vi "PCS-home.vi"() -> (3 "Stop":bool)   [LabVIEW 2011]
uses:
  <vilib>/Analysis/2dsp.llb/Integral Method.ctl
  <vilib>/Analysis/NI_AALPro.lvlib
  <vilib>/ptbypt/NI_PtbyPt.lvlib
  <vilib>/Analysis/NI_AALBase.lvlib
panel:
  out "Pfit":dbl
  out "Pcin":dbl(slide) scale=0.0..20.0 scale format="%#_2g"
  out "RTD-chamber (ºC)":sgl format="%0.2f"
  out "RTD-01 (ºC)":sgl format="%0.2f"
  out "RTD-02 (ºC)":sgl format="%0.2f"
  out "estado":bool
  out "slop":bool
  out "descarga 2":bool=TRUE
  out "time-loop":dbl
  in  "clear sample":bool
  out "cont_vacuo 2":u32[](array[numeric])
  out "Numeric":dbl
  out "Volume File":string
  out "Isotherm File":string
  in  "PCS":bool
  out "pathISO":path
  out "pathVV":path
  in  "Vertical Pause Button":bool
  out "tempo":dbl[](array[numeric])
  out "tempo 2":dbl[](array[numeric])
  out "output array":dbl[][](array[numeric])
  in  "T Ctrl":bool
  out "graph_completo":dynamicdata(graph)
  out "Vol02":dbl(slide) scale=0.0..20.0 scale format="%#_2g"
  out "Chamber":dbl(slide) scale=0.0..20.0 scale format="%#_2g"
  out "Vol01":dbl(slide) scale=0.0..20.0 scale format="%#_2g"
  in  "Tab Control":T1(tab)
  in  "Save As":bool
  out "path":path
  out "File name":string
  in  "Sample name":string
  in  "Nota 01":string
  in  "Open Button":bool
  out "stripped path":path
  in  "New file":string
  in  "array":dbl[](array[numeric])
  in  "SetP Array":bool
  in  "Npoint 2":i32
  in  "Pmax 2":i32
  out "Inter P 2":dbl
  out "Set ISO":dbl
  out "set P ISO":dbl
  in  "ISO Start":bool
  out "Inter P":dbl
  in  "Pmax":i32
  in  "Npoint":i32
  out "Set v v":dbl
  out "set P":dbl
  in  "V V Start":bool
  in  "Pressure Max":dbl
  in  "N cycles":dbl
  in  "Ch Max":bool
  in  "Save Discharge":bool
  out "Set ChM":dbl
  out "Cycles":dbl
  in  "Kinetic Save":bool
  out "slop01":T2(graph)
  out "fit-all":T3(graph)
  in  "SP-vol-01":dbl
  in  "command":string
  out "Abrir Gas":bool
  out "time (min)":dbl
  in  "Mininum Slope":dbl format="%#_6p"
  in  "total Time(min)":dbl
  in  "dp/dt min":dbl
  out "dp/dt":dbl format="%0.2f"
  out "slope":dbl format="%#_2p"
  out "time":dbl
  in  "t-vacuo (s)":dbl=1000.0
  in  "dp/dt min 2":dbl
  out "time (min) 2":dbl
  out "dp/dt 2":dbl format="%0.2f"
  in  "total Time(min) 2":dbl
  in  "Mininum Slope 2":dbl format="%#_6p"
  out "fit-all 2":T3(graph)
  out "slop01 2":T2(graph)
  out "slope 2":dbl format="%#_2p"
  out "vacuo (mBar)":dbl(knob) scale=0.0..20.0
  out "N 1bar":i32
  in  "t-vacuo (s) clean":dbl=1000.0
  out "time 3":dbl
  in  "New Button":bool
  out "Waveform T":dynamicdata(graph)
  out "ThermC":dbl(slide) scale=0.0..150.0
  in  "Ndata":i32
  in  "SP":dbl(slide) scale=0.0..150.0
  out "D-mean":dbl format="%0.2f"
  out "I-mean":dbl format="%0.2f"
  out "intrp- T":dbl format="%0.2f"
  out "min":dbl
  out "Max":dbl
  in  "PIDmin":dbl
  in  "PIDMax":dbl
  in  "PID":bool
  out "Ganho":dbl
  in  "Kp":dbl(slide) scale=0.0..10.0
  in  "D (Td)":bool
  in  "Kd(s)":dbl(slide) scale=0.0..10.0
  in  "I (Ti)":bool
  in  "Ki(s)":dbl(slide) scale=0.0..10.0
  out "milisec":dbl
  in  "fator Ganho":dbl=1.0
  out "t-on":dbl
  out "t-PID":bool
  in  "time (s) Loop":dbl
  in  "T - ON/OFF":bool
  in  "PID-ON/OFF":bool
  out "PID limit":bool
  in  "PID limit 2":dbl
  out "pause":bool
  in  "X time Off":dbl
  out "milisec 2":dbl
  out "ON/OFF":bool
  in  "close All":bool
  out "cont_desc":dbl[](array[numeric])
  out "Pvol2":dbl[](array[numeric])
  out "time 2":dbl[](array[numeric])
  out "cont_desc min":dbl[](array[numeric])
  out "Pvol2 total":dbl[](array[numeric])
  out "time (min) 3":dbl[](array[numeric])
  out "dP/dt":dbl[](array[numeric])
  out "x >= y? 2":bool
  out "cont_vacuo":u32[](array[numeric])
  out "PCv1":dbl[](array[numeric])
  out "t carga":dbl[](array[numeric])
  out "count":u32[](array[numeric])
  out "x >= y?":bool
  out "count 2":u32[](array[numeric])
  out "t completo":dbl[](array[numeric])
  out "PCv1 completo":dbl[](array[numeric])
  out "derivada 2":dbl[](array[numeric]) format="%#_4p"
  in  "initialize":bool
  out "SlopArray":dbl[](array[numeric]) format="%#_3p"
  out "cont":dbl[](array[numeric]) format="%#_6p"
  out "size(s)":i32
  in  "cargas-vol1":dbl
  in  "Discharge":bool
  in  "Charge":bool
  in  "stop":bool
  # "PCS - Pressure cycling system"
  # "Sorption isotherm"
  # "Maximum Charge"
  # "Void Volume"
  # "PID controller"
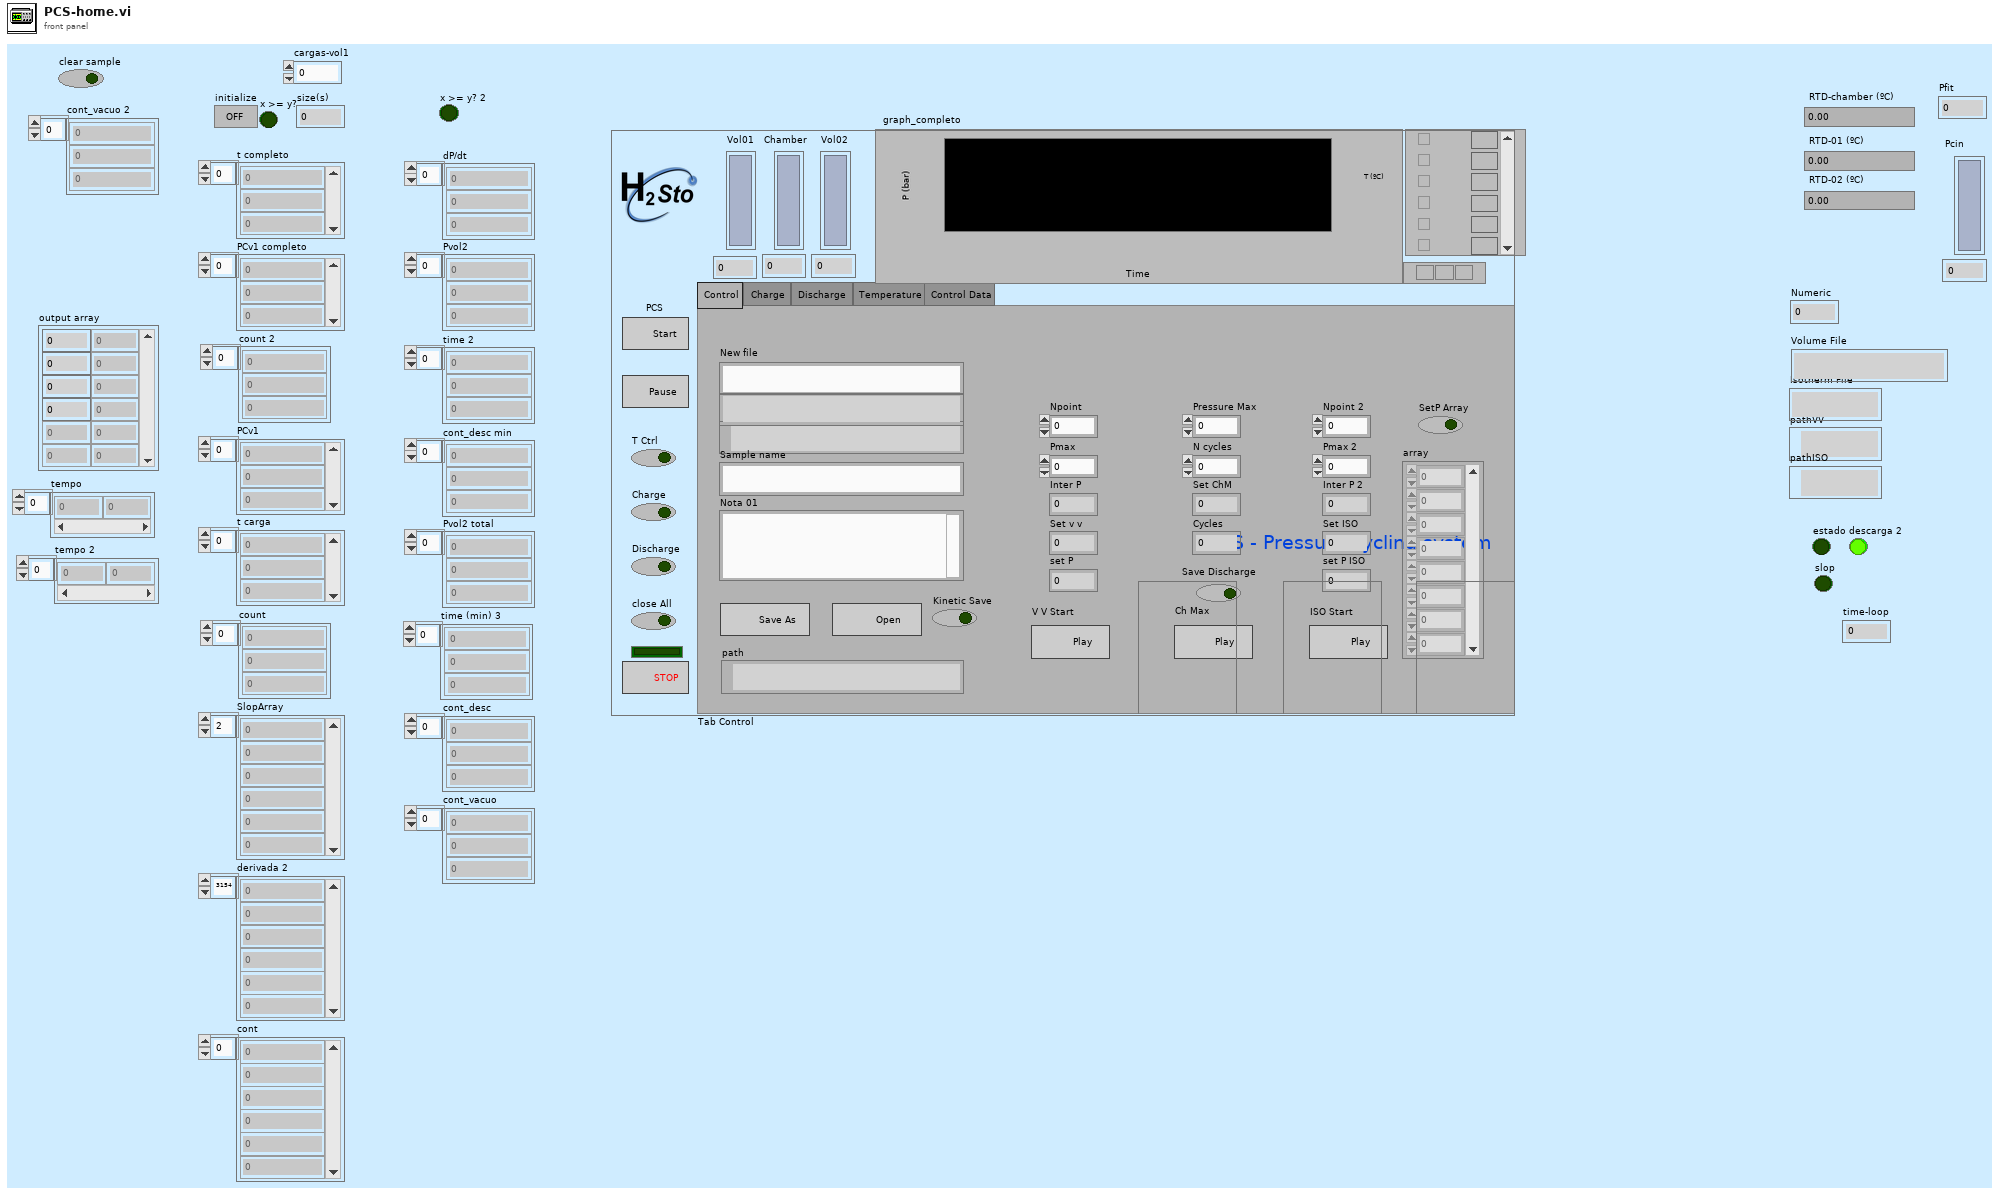
[diagram p1: front panel]
types:
  T1 = enum32{"Control", "Charge ", "Discharge ", "Temperature", "Control Data"}
  T2 = cluster{"Value":dbl[], "Best Linear Fit":dbl[]}[]
  T3 = cluster{"Value":dbl[], "Best Polynomial Fit":dbl[]}[]
  T4 = enum16{"open", "replace", "create", "open or create", "replace or create", "replace or create with confirmation"}
  T5 = enum16{"Linear", "Polynomial", "Spline", "Rational"}
  T6 = cluster{"Type of Interpolation":enum16{"Linear", "Polynomial", "Spline", "Rational"}, "Points Between":i32}
  T7 = typedef "NI_AALPro.lvlib/Integral Method.ctl" = i32
  T8 = cluster{"Value":dbl[], "Best Polynomial Fit":dbl[]}
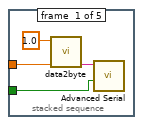
[diagram p2: hidden frame]
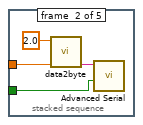
[diagram p3: hidden frame]
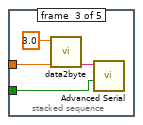
[diagram p4: hidden frame]
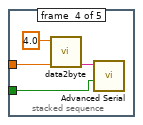
[diagram p5: hidden frame]
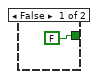
[diagram p6: hidden frame]
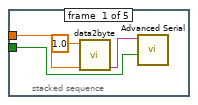
[diagram p8: hidden frame]
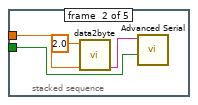
[diagram p9: hidden frame]
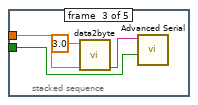
[diagram p10: hidden frame]
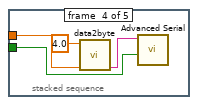
[diagram p11: hidden frame]
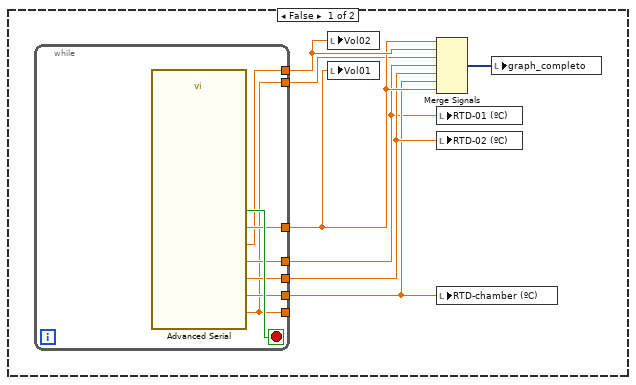
[diagram p12: hidden frame]
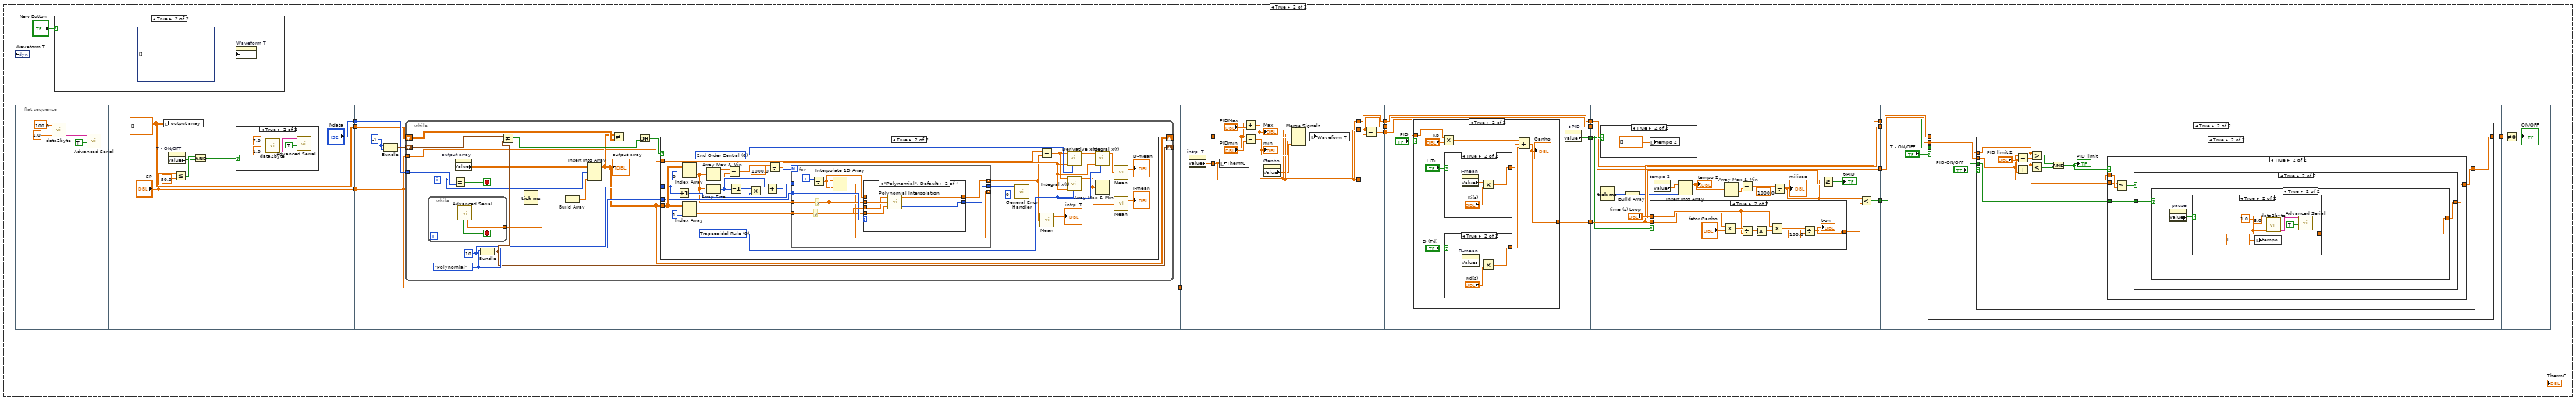
[diagram p13: hidden frame]
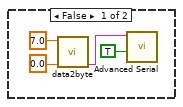
[diagram p15: hidden frame]
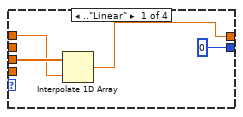
[diagram p17: hidden frame]
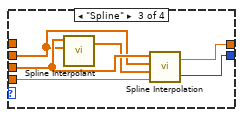
[diagram p18: hidden frame]
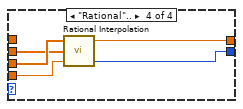
[diagram p19: hidden frame]
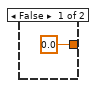
[diagram p20: hidden frame]
diagram:
  w1 = FALSE ("PCS")
  w8 = 1.0 ("Set ChM")
  n1 = while {
    stop <- w46 stop-if-true
    n2 = flat-sequence {
      tunnel: [w1623] -> w54
      tunnel: [w1622] -> w53
      tunnel: [w1618] -> w52
      tunnel: [w1621] -> w51
      tunnel: w54 -> [w1669]
      tunnel: w53 -> [w1668]
      tunnel: w52 -> [w1667]
      tunnel: w51 -> [w1659]
      frame #0 {
        n3 = case shown="True" "Save As" {
          selector: "Save As" -> [_ w1646]
          tunnel: [w1642 w1647] -> w1624
          tunnel: [FALSE w1646] -> w1623
          frame False {
            n4 = property on="path" class="Path"() -> ("Value"=w1642:path)  [unwired: 2 in, 2 out]
          }
          frame True {
            n5 = call "data_file.vi"("Nota 01"="Nota 01", "Sample name"="Sample name", "File name"="New file") -> ("path"=w1647:path)  [unwired: 8 in]
          }
        }
        n6 = local write "path"(w1624) -> ()
        n7 = Strip Path(path=w1624) -> (stripped path=w1620:path, name=w1619:string)
        "stripped path" <- w1620
        n8 = local write "File name"(w1619) -> ()
        n9 = case shown="True" "Open Button" {
          selector: "Open Button" -> [_ w1632]
          tunnel: [FALSE w1632] -> w1622
          tunnel: [w1628 w1631] -> w1621
          tunnel: w1620 -> [w1628 _]
          tunnel: [w1627 w1630] -> w1618
          tunnel: w1619 -> [w1627 _]
          frame False {
          }
          frame True {
            n10 = File Dialog(6:"*.txt" ("pattern label")) -> (0:w1636:errorcluster, 3:w1635:path)  [unwired: 3 in, 5 out]
            n11 = Open/Create/Replace File(file path (use dialog)=w1635, error in=w1636, operation (0:open)=T4."open", access (0:read/write)=enum16{"read/write", "read-only", "write-only"}."read/write") -> (refnum out=w1638:refnum<file>, error out=w1637:errorcluster)  [unwired: 2 in, 1 out]
            n12 = Close File(refnum=w1638, error in=w1637) -> (path=w1634:path)  [unwired: 1 out]
            n13 = local write "path"(w1634) -> ()
            n14 = Strip Path(path=w1634) -> (stripped path=w1631:path, name=w1630:string)
            n15 = local write "stripped path"(w1631) -> ()
            n16 = local write "File name"(w1630) -> ()
          }
        }
      }
      frame #1 {
        w1649 = "\t"
        w1661 = "\t"
        n17 = Or(x=w1669, y=w1668) -> (x .or. y?=w1670:bool)
        n18 = Concatenate Strings("set" ("search string/char (-)"), w1661, "Pv1" ("search string/char (-)"), w1661, "Pc" ("search string/char (-)"), w1661, "Tv1" ("search string/char (-)"), w1661, "Tc" ("search string/char (-)")) -> (w1651:string)
        n19 = Concatenate Strings("Cycle" ("search string/char (-)"), w1649, "set" ("search string/char (-)"), w1649, "Pit(vol1)" ("search string/char (-)"), w1649, "Pf2(Pc)" ("search string/char (-)"), w1649, "ZPf2(Pv2)" ("search string/char (-)"), w1649, "T1" ("search string/char (-)"), w1649, "Tc" ("search string/char (-)"), w1649, "T2" ("search string/char (-)")) -> (w1650:string)
        n20 = property on="path" class="Path"() -> ("Value"=w1666:path)  [unwired: 2 in, 2 out]
        n21 = case shown="True" w1670 {
          tunnel: w1667 -> [_ w1690]
          tunnel: w1659 -> [_ w1689]
          tunnel: w1666 -> [_ w1684]
          tunnel: w1651 -> [_ w1675]
          tunnel: w1650 -> [_ w1672]
          frame False {
          }
          frame True {
            n22 = flat-sequence {
              tunnel: w1689 -> [w1699]
              tunnel: w1690 -> [w1700]
              tunnel: [w1700] -> w1688
              tunnel: [w1699] -> w1687
              tunnel: w1684 -> [w1693]
              tunnel: [w1694] -> w1683
              tunnel: [w1693] -> w1681
              tunnel: w1675 -> [w1692]
              tunnel: [w1692] -> w1674
              tunnel: [w1691] -> w1673
              tunnel: w1672 -> [w1691]
              tunnel: w1688 -> [w1729]
              tunnel: w1687 -> [w1715]
              tunnel: [w1724] -> w1686
              tunnel: [w1723] -> w1685
              tunnel: w1683 -> [w1704]
              tunnel: [w1726] -> w1682
              tunnel: w1681 -> [w1725]
              tunnel: [w1725] -> w1680
              tunnel: [w1709] -> w1677
              tunnel: [w1708] -> w1676
              tunnel: w1674 -> [w1703]
              tunnel: w1673 -> [w1702]
              tunnel: [w1701] -> w1671
              tunnel: w1686 -> [w1744]
              tunnel: w1685 -> [w1743]
              tunnel: w1682 -> [w1742]
              tunnel: w1680 -> [w1741]
              tunnel: [w1741] -> w1679
              tunnel: w1677 -> [w1736]
              tunnel: w1676 -> [w1735]
              tunnel: w1671 -> [w1734]
              tunnel: w1679 -> [w1747]
              tunnel: [w1747] -> w1678
              tunnel: w1678 -> [w1767]
              frame #0 {
                n23 = Open/Create/Replace File(file path (use dialog)=w1693) -> (refnum out=w1697:refnum<file>, error out=w1698:errorcluster)  [unwired: 5 in, 1 out]
                n24 = Read from Text File(file (use dialog)=w1697, error in=w1698) -> (refnum out=w1695:refnum<file>, text=w1694:string, error out=w1696:errorcluster)  [unwired: 2 in, 1 out]
                n25 = Close File(refnum=w1695, error in=w1696) -> ()  [unwired: 2 out]
              }
              frame #1 {
                w1705 = "\r"
                w1710 = enum16{"start", "end", "current"}."end" ("from (0:start)")
                w1728 = "\r"
                w1711 = T4."replace or create with confirmation" ("operation (0:open)")
                n26 = Search/Split String(string=w1729, search string/char (-)=".txt") -> (substring before match=w1717:string, match + rest of string=w1718:string)  [unwired: 1 in, 1 out]
                n27 = Concatenate Strings(w1717, "_vv" ("search string/char (-)"), w1718) -> (w1731:string)
                "Volume File" <- w1731
                n28 = Concatenate Strings(w1717, "_iso" ("search string/char (-)"), w1718) -> (w1716:string)
                "Isotherm File" <- w1716
                n29 = Build Path(base path=w1715, name or relative path=w1731) -> (appended path=w1730:path)
                n30 = Build Path(base path=w1715, name or relative path=w1716) -> (appended path=w1712:path)
                n31 = Concatenate Strings(w1728, w1704, "============" ("search string/char (-)"), w1728, w1703, "\r\n") -> (w1726:string)
                n32 = Concatenate Strings(w1705, w1704, "============" ("search string/char (-)"), w1705, w1702, "\r\n") -> (w1701:string)
                n33 = Open/Create/Replace File(file path (use dialog)=w1730, operation (0:open)=w1711) -> (refnum out=w1722:refnum<file>, error out=w1721:errorcluster)  [unwired: 4 in, 1 out]
                n34 = Open/Create/Replace File(file path (use dialog)=w1712, operation (0:open)=w1711) -> (refnum out=w1713:refnum<file>, error out=w1714:errorcluster)  [unwired: 4 in, 1 out]
                n35 = Set File Position(refnum=w1722, from (0:start)=w1710, error in=w1721) -> (refnum out=w1724:refnum<file>, error out=w1723:errorcluster)  [unwired: 1 in]
                n36 = Set File Position(refnum=w1713, from (0:start)=w1710, error in=w1714) -> (refnum out=w1709:refnum<file>, error out=w1708:errorcluster)  [unwired: 1 in]
              }
              frame #2 {
                n37 = Write to Text File(file (use dialog)=w1744, text=w1742, error in=w1743) -> (refnum out=w1746:refnum<file>, error out=w1745:errorcluster)  [unwired: 1 in, 1 out]
                n38 = Write to Text File(file (use dialog)=w1736, text=w1734, error in=w1735) -> (refnum out=w1737:refnum<file>, error out=w1738:errorcluster)  [unwired: 1 in, 1 out]
                n39 = Close File(refnum=w1746, error in=w1745) -> (path=→"pathVV":path)  [unwired: 1 out]
                n40 = Close File(refnum=w1737, error in=w1738) -> (path=→"pathISO":path)  [unwired: 1 out]
              }
              frame #3 {
              }
              frame #4 {
                w1766 = "\t"
                n41 = Open/Create/Replace File(file path (use dialog)=w1767, access (0:read/write)=enum16{"read/write", "read-only", "write-only"}."write-only") -> (refnum out=w1755:refnum<file>, error out=w1751:errorcluster)  [unwired: 4 in, 1 out]
                n42 = Set File Position(refnum=w1755, from (0:start)=enum16{"start", "end", "current"}."end", error in=w1751) -> (refnum out=w1754:refnum<file>, error out=w1753:errorcluster)  [unwired: 1 in]
                n43 = Concatenate Strings("============" ("search string/char (-)"), "\r", "Date-time" ("search string/char (-)"), w1766, "Pv1" ("search string/char (-)"), w1766, "Pc" ("search string/char (-)"), w1766, "Pv2" ("search string/char (-)"), w1766, "T1" ("search string/char (-)"), w1766, "Tc" ("search string/char (-)"), w1766, "T2" ("search string/char (-)"), w1766, "Pcin" ("search string/char (-)"), "\r\n") -> (w1758:string)
                n44 = Write to Text File(file (use dialog)=w1754, text=w1758, error in=w1753) -> (refnum out=w1768:refnum<file>, error out=w1769:errorcluster)  [unwired: 1 in, 1 out]
                n45 = Close File(refnum=w1768, error in=w1769) -> ()  [unwired: 2 out]
              }
            }
          }
        }
      }
    }
    n46 = property class="VI"() -> (error out=w56:errorcluster, "Front Panel"=w57:refnum<vi>)  [unwired: 2 in, 1 out]
    n47 = flat-sequence {
      tunnel: [w1471] -> w45
      frame #0 {
        n48 = case shown="True" "Kinetic Save" {
          frame False {
            n49 = while {
              tunnel: [w100] -> w92
              tunnel: [w95] -> w89
              tunnel: [w99] -> w93
              tunnel: [w97] -> w88
              tunnel: [w96] -> w91
              tunnel: [w98] -> w90
              tunnel: [w95] -> _
              stop <- w101 stop-if-true
              n50 = call "Advanced Serial.vi"() -> ("RTD-02 (ºC)"=w96:sgl, "RTD-01 (ºC)"=w97:sgl, "vacuo (mBar)"=w95:dbl, "P02 (Bar)"=w99:dbl, "RTD-chamber (ºC)"=w98:sgl, "P01 (Bar)"=w100:dbl, "32bytes"=w101:bool)  [unwired: 5 in]
            }
            n51 = local write "Vol02"(w93) -> ()
            n52 = local write "Vol01"(w92) -> ()
            n53 = Merge Signals(w92, w93, w89, w88, w91, w90, w92) -> (w94:dynamicdata)
            n54 = local write "RTD-01 (ºC)"(w88) -> ()
            n55 = local write "RTD-02 (ºC)"(w91) -> ()
            n56 = local write "RTD-chamber (ºC)"(w90) -> ()
            n57 = local write "graph_completo"(w94) -> ()
          }
          frame True {
            w113 = "\t"
            w110 = i16 4 ("precision (6)")
            n58 = while {
              tunnel: [w131] -> w107
              tunnel: [w130] -> w106
              tunnel: [w129] -> w104
              tunnel: [w127] -> w102
              tunnel: [w128] -> w103
              tunnel: [w126] -> w105
              stop <- w132 stop-if-true
              n59 = call "Advanced Serial.vi"() -> ("RTD-02 (ºC)"=w128:sgl, "RTD-01 (ºC)"=w129:sgl, "vacuo (mBar)"=w126:dbl, "P02 (Bar)"=w130:dbl, "RTD-chamber (ºC)"=w127:sgl, "P01 (Bar)"=w131:dbl, "32bytes"=w132:bool)  [unwired: 5 in]
            }
            n60 = property on="Pcin" class="Slide (strict)"() -> ("Value"=w109:dbl)  [unwired: 2 in, 2 out]
            n61 = Number To Fractional String(number=w109, precision (6)=w110) -> (F-format string=w111:string)  [unwired: 2 in]
            n62 = local write "Vol01"(w107) -> ()
            n63 = local write "Vol02"(w106) -> ()
            n64 = Number To Fractional String(number=w107, precision (6)=w110) -> (F-format string=w122:string)  [unwired: 2 in]
            n65 = Merge Signals(w107, w106, w105, w104, w103, w102, w107) -> (w108:dynamicdata)
            n66 = Number To Fractional String(number=w106, precision (6)=w110) -> (F-format string=w121:string)  [unwired: 2 in]
            n67 = Number To Fractional String(number=w104, precision (6)=w110) -> (F-format string=w119:string)  [unwired: 2 in]
            n68 = local write "RTD-01 (ºC)"(w104) -> ()
            n69 = local write "RTD-02 (ºC)"(w103) -> ()
            n70 = Number To Fractional String(number=w103, precision (6)=w110) -> (F-format string=w117:string)  [unwired: 2 in]
            n71 = Number To Fractional String(number=w102, precision (6)=w110) -> (F-format string=w118:string)  [unwired: 2 in]
            n72 = local write "RTD-chamber (ºC)"(w102) -> ()
            n73 = local write "graph_completo"(w108) -> ()
            n74 = Get Date/Time String(want seconds? (F)=TRUE) -> (date string=w125:string, time string=w123:string)  [unwired: 2 in]
            n75 = Concatenate Strings(w125, "-" ("string"), w123, w113, w122, w113, "-" ("string"), w113, w121, w113, w119, w113, w118, w113, w117, w113, w111, "\r\n") -> (w116:string)
            n76 = property on="path" class="Path"() -> ("Value"=w115:path)  [unwired: 2 in, 2 out]
            n77 = call "write_file.vi"("text"=w116, "file path (use dialog)"=w115) -> ()  [unwired: 10 in]
          }
        }
      }
      frame #1 {
        n78 = case shown="False" "T Ctrl" {
          frame False {
          }
          frame True {
            n79 = flat-sequence {
              tunnel: ["SP"] -> w155
              tunnel: ["Ndata"] -> w154
              tunnel: [w166] -> w153
              tunnel: w155 -> [w176]
              tunnel: [w176] -> w152
              tunnel: w154 -> [w178]
              tunnel: w153 -> [w177]
              tunnel: w152 -> [w260]
              tunnel: [w260] -> w151
              tunnel: [w259] -> w150
              tunnel: w151 -> [w263]
              tunnel: w150 -> [w262]
              tunnel: [w262] -> w149
              tunnel: [w263] -> w148
              tunnel: [w262] -> w147
              tunnel: w149 -> [w271]
              tunnel: w148 -> [w270]
              tunnel: [w270] -> w146
              tunnel: [w272] -> w145
              tunnel: [w269] -> w144
              tunnel: w147 -> [w269]
              tunnel: w146 -> [w278]
              tunnel: [w278] -> w143
              tunnel: w145 -> [w276]
              tunnel: [w275] -> w142
              tunnel: [w274] -> w141
              tunnel: [w273] -> w140
              tunnel: w144 -> [w273]
              tunnel: w143 -> [w312]
              tunnel: [w312] -> w139
              tunnel: w142 -> [w308]
              tunnel: [w308] -> w138
              tunnel: [w307] -> w137
              tunnel: w141 -> [w297]
              tunnel: [w296] -> w136
              tunnel: w140 -> [w296]
              tunnel: w139 -> [w327]
              tunnel: w138 -> [_]
              tunnel: w137 -> [w326]
              tunnel: w136 -> [w325]
              tunnel: [w324] -> w135
              tunnel: w135 -> [w409]
              frame #0 {
                n80 = call "data2byte.vi"("argument"=1.0 ("number"), "new function"=100.0) -> ("protocol"=w157:string)  [unwired: 8 in, 1 out]
                n81 = call "Advanced Serial.vi"("Write"=TRUE ("write"), "string to write"=w157) -> ()  [unwired: 3 in, 7 out]
              }
              frame #1 {
                w166 = dbl[][] [] ("Array 2")
                n82 = local write "output array"(w166) -> ()
                n83 = property on="T - ON/OFF" class="Bool (strict)"() -> ("Value"=w161:bool)  [unwired: 2 in, 2 out]
                n84 = Less Or Equal?(x="SP", y=50.0) -> (x <= y?=w162:bool)
                n85 = And(x=w162, y=w161) -> (x .and. y?=w163:bool)
                n86 = case shown="True" w163 {
                  frame False {
                    n87 = call "data2byte.vi"("argument"=0.0 ("number"), "new function"=7.0) -> ("protocol"=w168:string)  [unwired: 8 in, 1 out]
                    n88 = call "Advanced Serial.vi"("Write"=TRUE ("write"), "string to write"=w168) -> ()  [unwired: 3 in, 7 out]
                  }
                  frame True {
                    n89 = call "data2byte.vi"("argument"=1.0 ("number"), "new function"=7.0) -> ("protocol"=w172:string)  [unwired: 8 in, 1 out]
                    n90 = call "Advanced Serial.vi"("Write"=TRUE ("write"), "string to write"=w172) -> ()  [unwired: 3 in, 7 out]
                  }
                }
              }
              frame #2 {
                w179 = -1
                n91 = Bundle(w179, w179) -> (w180:cluster{i32, i32})  [unwired: 1 in]
                n92 = while {
                  shift-left: w180 -> [w192]
                  shift-right: [w191] -> _
                  shift-left: w177 -> [w197]
                  shift-right: [w188] -> _
                  tunnel: w178 -> [w184]
                  tunnel: w176 -> [w182]
                  i -> [w183]
                  stop <- w185 stop-if-true
                  w190 = 10 ("Points Between")
                  w193 = T5."Polynomial" ("Type of Interpolation")
                  n93 = while {
                    tunnel: [w198] -> w186
                    stop <- w199 stop-if-true
                    n94 = call "Advanced Serial.vi"() -> ("RTD-chamber (ºC)"=w198:sgl, "32bytes"=w199:bool)  [unwired: 5 in, 5 out]
                  }
                  n95 = Equal?(x=w183, y=w184) -> (x = y?=w185:bool)
                  n96 = property on="output array" class="Arr (strict)"() -> ("Value"=w187:dbl[][])  [unwired: 2 in, 2 out]
                  n97 = Bundle("Type of Interpolation"=w193, "Points Between"=w190) -> (w191:T6)  [unwired: 1 in]
                  n98 = Not Equal?(x=w192, y=w191) -> (x != y?=w195:bool)
                  n99 = Tick Count (ms)() -> (millisecond timer value=w181:u32)
                  n100 = Build Array(w181, w186) -> (w189:sgl[])
                  n101 = Insert Into Array(array=w187, index (row)=w183, new element=w189) -> (w188:dbl[][])  [unwired: 1 in]
                  "output array" <- w188
                  n102 = Not Equal?(x=w188, y=w197) -> (x != y?=w196:bool)
                  n103 = Or(x=w196, y=w195) -> (x .or. y?=w194:bool)
                  n104 = case shown="True" w194 {
                    tunnel: w188 -> [_ w225]
                    tunnel: w193 -> [_ w219]
                    tunnel: w190 -> [_ w218]
                    tunnel: w182 -> [_ w215]
                    frame False {
                    }
                    frame True {
                      w210 = T7 0 items=["Trapezoidal Rule", "Simpson's Rule", "Simpson's 3/8 Rule", "Bode Rule"] ("integration method")
                      w216 = u16 0 items=["2nd Order Central", "4th Order Central", "Forward", "Backward"] ("method")
                      n105 = Increment(x=w218) -> (x+1=w223:i32)
                      n106 = Index Array(array=w225, index (col)=0) -> (element=w209:dbl[])  [unwired: 1 in]
                      n107 = Index Array(array=w225, index (col)=1) -> (element=w204:dbl[])  [unwired: 1 in]
                      n108 = Array Max & Min(array=w209) -> (max value=w213:dbl, min value=w212:dbl)  [unwired: 2 out]
                      n109 = Array Size(array=w209) -> (size(s)=w221:i32)
                      n110 = Subtract(x=w213, y=w212) -> (x-y=w202:dbl)
                      n111 = Decrement(x=w221) -> (x-1=w224:i32)
                      n112 = Multiply(x=w224, y=w218) -> (x*y=w222:i32)
                      n113 = Add(x=w221, y=w222) -> (x+y=w220:i32)
                      n114 = Divide(x=w202, y=1000.0) -> (x/y=w201:dbl)
                      n115 = for {
                        N: w220 -> [_]
                        tunnel: w204 -> [w238]
                        tunnel: w209 -> [w232]
                        tunnel: [w237] -> w229
                        tunnel: w219 -> [w233]
                        tunnel: w223 -> [w235]
                        tunnel: [w234] -> w200 mode=indexing
                        tunnel: [w231] -> _ mode=indexing
                        i -> [w236]
                        # "x"
                        # "y"
                        n116 = Divide(x=w236, y=w235) -> (x/y=w230:dbl)
                        n117 = Interpolate 1D Array(1:w230, 2:w232) -> (0:w231:dbl)
                        n118 = case shown="\"Polynomial\", Default" w233 {
                          tunnel: w231 -> [_ w247 w250 w254]
                          tunnel: [w241 w246 w248 w256] -> w234
                          tunnel: [0 w245 w249 w255] -> w237
                          tunnel: w232 -> [_ w244 w251 w257]
                          tunnel: w238 -> [w242 w243 w253 w258]
                          tunnel: w230 -> [w239 _ _ _]
                          frame .."Linear" {
                            n119 = Interpolate 1D Array(1:w239, 2:w242) -> (0:w241:dbl)
                          }
                          frame "Polynomial", Default {
                            n120 = call <vilib>:"Polynomial Interpolation.vi"("x value"=w247, "X"=w244, "Y"=w243) -> ("error"=w245:i32, "interpolation value"=w246:dbl)  [unwired: 1 out]
                          }
                          frame "Spline" {
                            n121 = call <vilib>:"Spline Interpolant.vi"("X"=w251, "Y"=w253) -> ("Interpolant"=w252:dbl[])  [unwired: 2 in, 1 out]
                            n122 = call <vilib>:"Spline Interpolation.vi"("x value"=w250, "Interpolant"=w252, "X"=w251, "Y"=w253) -> ("error"=w249:i32, "interpolation value"=w248:dbl)
                          }
                          frame "Rational".. {
                            n123 = call <vilib>:"Rational Interpolation.vi"("x value"=w254, "X"=w257, "Y"=w258) -> ("error"=w255:i32, "interpolation value"=w256:dbl)  [unwired: 1 out]
                          }
                        }
                      }
                      n124 = call <vilib>:"General Error Handler.vi"("[error code] (0)"=w229, "type of dialog (OK msg:1)"=0) -> ()  [unwired: 9 in, 5 out]
                      n125 = Subtract(x=w215, y=w200) -> (x-y=w214:dbl[])
                      n126 = call <vilib>:"Mean.vi"("X"=w200) -> ("mean"=→"intrp- T":dbl)  [unwired: 1 out]
                      n127 = call <vilib>:"Derivative x(t).vi"("method"=w216, "dt"=w201, "X"=w214) -> ("dX/dt"=w211:dbl[])  [unwired: 7 in, 1 out]
                      n128 = call <vilib>:"Integral x(t).vi"("integration method"=w210, "dt"=w201, "X"=w214) -> ("Integral X"=w205:dbl[])  [unwired: 7 in, 1 out]
                      n129 = call <vilib>:"Integral x(t).vi"("integration method"=w210, "dt"=w201, "X"=w211) -> ("Integral X"=w208:dbl[])  [unwired: 7 in, 1 out]
                      n130 = Array Max & Min(array=w205) -> ()  [unwired: 4 out]
                      n131 = call <vilib>:"Mean.vi"("X"=w208) -> ("mean"=→"D-mean":dbl)  [unwired: 1 out]
                      n132 = call <vilib>:"Mean.vi"("X"=w205) -> ("mean"=→"I-mean":dbl)  [unwired: 1 out]
                    }
                  }
                }
              }
              frame #3 {
                n133 = property on="intrp- T" class="DigNum (strict)"() -> ("Value"=w259:dbl)  [unwired: 2 in, 2 out]
              }
              frame #4 {
                n134 = local write "ThermC"(w262) -> ()
                n135 = Add(x=w263, y="PIDMax") -> (x+y=w264:dbl)
                "Max" <- w264
                n136 = Subtract(x=w263, y="PIDmin") -> (x-y=w265:dbl)
                "min" <- w265
                n137 = property on="Ganho" class="DigNum (strict)"() -> ("Value"=w261:dbl)  [unwired: 2 in, 2 out]
                n138 = Merge Signals(w263, w262, w264, w265, w261) -> (w266:dynamicdata)
                n139 = local write "Waveform T"(w266) -> ()
              }
              frame #5 {
                n140 = Subtract(x=w270, y=w271) -> (x-y=w272:dbl)
              }
              frame #6 {
                n141 = case shown="True" "PID" {
                  tunnel: w276 -> [_ w281]
                  tunnel: [0.0 w280] -> w275
                  frame False {
                  }
                  frame True {
                    n142 = Multiply(x=w281, y="Kp") -> (x*y=w284:dbl)
                    n143 = case shown="True" "I (Ti)" {
                      tunnel: [0.0 w295] -> w283
                      frame False {
                      }
                      frame True {
                        n144 = property on="I-mean" class="DigNum (strict)"() -> ("Value"=w293:dbl)  [unwired: 2 in, 2 out]
                        n145 = Multiply(x=w293, y="Ki(s)") -> (x*y=w295:dbl)
                      }
                    }
                    n146 = case shown="True" "D (Td)" {
                      tunnel: [0.0 w291] -> w282
                      frame False {
                      }
                      frame True {
                        n147 = property on="D-mean" class="DigNum (strict)"() -> ("Value"=w289:dbl)  [unwired: 2 in, 2 out]
                        n148 = Multiply(x=w289, y="Kd(s)") -> (x*y=w291:dbl)
                      }
                    }
                    n149 = Compound Arithmetic op=ADD(w284, w283, w282) -> (w280:dbl)
                    "Ganho" <- w280
                  }
                }
                n150 = property on="t-PID" class="Bool (strict)"() -> ("Value"=w274:bool)  [unwired: 2 in, 2 out]
              }
              frame #7 {
                n151 = case shown="True" w297 {
                  frame False {
                  }
                  frame True {
                    n152 = local write "tempo 2"(dbl[] [] ("Time")) -> ()
                  }
                }
                n153 = Tick Count (ms)() -> (millisecond timer value=w304:u32)
                n154 = Build Array(w304) -> (w305:u32[])
                n155 = case shown="True" w297 {
                  tunnel: w308 -> [_ w323]
                  tunnel: "time (s) Loop" -> [_ w320]
                  tunnel: [w314 w317] -> w309
                  frame False {
                    n156 = property on="t-on" class="DigNum (strict)"() -> ("Value"=w314:dbl)  [unwired: 2 in, 2 out]
                  }
                  frame True {
                    n157 = Multiply(x=w323, y="fator Ganho") -> (x*y=w322:dbl)
                    n158 = Divide(x=w322, y=w320) -> (x/y=w321:dbl)
                    n159 = Absolute Value(x=w321) -> (abs(x)=w319:dbl)
                    n160 = Multiply(x=w320, y=w319) -> (x*y=w318:dbl)
                    n161 = Divide(x=w318, y=100.0) -> (x/y=w317:dbl)
                    "t-on" <- w317
                  }
                }
                n162 = property on="tempo 2" class="Arr (strict)"() -> ("Value"=w306:dbl[])  [unwired: 2 in, 2 out]
                n163 = Insert Into Array(array=w306, new element=w305) -> (w303:dbl[])  [unwired: 1 in]
                "tempo 2" <- w303
                n164 = Array Max & Min(array=w303) -> (max value=w302:dbl, min value=w301:dbl)  [unwired: 2 out]
                n165 = Subtract(x=w302, y=w301) -> (x-y=w300:dbl)
                n166 = Divide(x=w300, y=1000.0) -> (x/y=w298:dbl)
                "milisec" <- w298
                n167 = Greater Or Equal?(x=w298, y="time (s) Loop") -> (x >= y?=→"t-PID":bool)
                n168 = Less?(x=w298, y=w309) -> (x < y?=w307:bool)
              }
              frame #8 {
                n169 = case shown="True" "T - ON/OFF" {
                  tunnel: w327 -> [_ w333]
                  tunnel: w326 -> [_ w332]
                  tunnel: w325 -> [_ w331]
                  tunnel: [0.0 ("number") w330] -> w324
                  frame False {
                  }
                  frame True {
                    n170 = case shown="True" "PID-ON/OFF" {
                      tunnel: w333 -> [w338 w355]
                      tunnel: w332 -> [_ w349]
                      tunnel: w331 -> [w337 w348]
                      tunnel: [w336 w347] -> w330
                      frame False {
                        n171 = Greater?(x=w338, y=w337) -> (0:w335:bool)
                        n172 = case shown="True" w335 {
                          tunnel: [w339 w343] -> w336
                          frame False {
                            w339 = 0.0 ("number")
                            n173 = call "data2byte.vi"("argument"=w339, "new function"=6.0) -> ("protocol"=w340:string)  [unwired: 8 in, 1 out]
                            n174 = call "Advanced Serial.vi"("Write"=TRUE ("write"), "string to write"=w340) -> ()  [unwired: 3 in, 7 out]
                          }
                          frame True {
                            w343 = 1.0 ("number")
                            n175 = call "data2byte.vi"("argument"=w343, "new function"=6.0) -> ("protocol"=w344:string)  [unwired: 8 in, 1 out]
                            n176 = call "Advanced Serial.vi"("Write"=TRUE ("write"), "string to write"=w344) -> ()  [unwired: 3 in, 7 out]
                          }
                        }
                      }
                      frame True {
                        n177 = Subtract(x=w355, y="PID limit 2") -> (x-y=w351:dbl)
                        n178 = Add(x=w355, y="PID limit 2") -> (x+y=w350:dbl)
                        n179 = Greater?(x=w348, y=w351) -> (0:w353:bool)
                        n180 = Less?(x=w348, y=w350) -> (x < y?=w352:bool)
                        n181 = And(x=w353, y=w352) -> (x .and. y?=w354:bool)
                        "PID limit" <- w354
                        n182 = case shown="True" w354 {
                          tunnel: w355 -> [w361 w374]
                          tunnel: w349 -> [_ w373]
                          tunnel: w348 -> [w359 w371]
                          tunnel: [w358 w370] -> w347
                          frame False {
                            n183 = Greater?(x=w361, y=w359) -> (0:w357:bool)
                            n184 = local write "t-on"(0.0 ("%t-on")) -> ()
                            n185 = case shown="True" w357 {
                              tunnel: [w362 w366] -> w358
                              frame False {
                                w362 = 0.0 ("number")
                                n186 = call "data2byte.vi"("argument"=w362, "new function"=6.0) -> ("protocol"=w363:string)  [unwired: 8 in, 1 out]
                                n187 = call "Advanced Serial.vi"("Write"=TRUE ("write"), "string to write"=w363) -> ()  [unwired: 3 in, 7 out]
                              }
                              frame True {
                                w366 = 1.0 ("number")
                                n188 = call "data2byte.vi"("argument"=w366, "new function"=6.0) -> ("protocol"=w367:string)  [unwired: 8 in, 1 out]
                                n189 = call "Advanced Serial.vi"("Write"=TRUE ("write"), "string to write"=w367) -> ()  [unwired: 3 in, 7 out]
                              }
                            }
                          }
                          frame True {
                            n190 = Less Or Equal?(x=w371, y=w374) -> (x <= y?=w372:bool)
                            n191 = case shown="True" w372 {
                              tunnel: [w375 w379] -> w370
                              tunnel: w373 -> [_ w380]
                              frame False {
                                w375 = 0.0 ("number")
                                n192 = call "data2byte.vi"("argument"=w375, "new function"=6.0) -> ("protocol"=w376:string)  [unwired: 8 in, 1 out]
                                n193 = call "Advanced Serial.vi"("Write"=TRUE ("write"), "string to write"=w376) -> ()  [unwired: 3 in, 7 out]
                              }
                              frame True {
                                n194 = case shown="True" w380 {
                                tunnel: [w381 w399] -> w379
                                frame False {
                                w381 = 0.0 ("number")
                                n195 = Tick Count (ms)() -> (millisecond timer value=w388:u32)
                                n196 = Build Array(w388) -> (w387:u32[])
                                n197 = property on="time (s) Loop" class="DigNum (strict)"() -> ("Value"=w396:dbl)  [unwired: 2 in, 2 out]
                                n198 = call "data2byte.vi"("argument"=w381, "new function"=6.0) -> ("protocol"=w384:string)  [unwired: 8 in, 1 out]
                                n199 = property on="tempo" class="Arr (strict)"() -> ("Value"=w386:dbl[])  [unwired: 2 in, 2 out]
                                n200 = call "Advanced Serial.vi"("Write"=TRUE ("write"), "string to write"=w384) -> ()  [unwired: 3 in, 7 out]
                                n201 = Multiply(x=w396, y="X time Off") -> (x*y=w395:dbl)
                                n202 = Insert Into Array(array=w386, new element=w387) -> (w389:dbl[])  [unwired: 1 in]
                                "tempo" <- w389
                                n203 = Array Max & Min(array=w389) -> (max value=w390:dbl, min value=w391:dbl)  [unwired: 2 out]
                                n204 = Subtract(x=w390, y=w391) -> (x-y=w392:dbl)
                                n205 = Divide(x=w392, y=1000.0) -> (x/y=w394:dbl)
                                "milisec 2" <- w394
                                n206 = Greater Or Equal?(x=w394, y=w395) -> (x >= y?=→"pause":bool)
                                }
                                frame True {
                                n207 = property on="pause" class="Bool (strict)"() -> ("Value"=w398:bool)  [unwired: 2 in, 2 out]
                                n208 = case shown="True" w398 {
                                tunnel: [w400 w404] -> w399
                                frame False {
                                w400 = 0.0 ("number")
                                n209 = call "data2byte.vi"("argument"=w400, "new function"=6.0) -> ("protocol"=w401:string)  [unwired: 8 in, 1 out]
                                n210 = call "Advanced Serial.vi"("Write"=TRUE ("write"), "string to write"=w401) -> ()  [unwired: 3 in, 7 out]
                                }
                                frame True {
                                w404 = 1.0 ("number")
                                n211 = local write "tempo"(dbl[] [] ("tempo")) -> ()
                                n212 = call "data2byte.vi"("argument"=w404, "new function"=6.0) -> ("protocol"=w405:string)  [unwired: 8 in, 1 out]
                                n213 = call "Advanced Serial.vi"("Write"=TRUE ("write"), "string to write"=w405) -> ()  [unwired: 3 in, 7 out]
                                }
                                }
                                }
                                }
                              }
                            }
                          }
                        }
                      }
                    }
                  }
                }
              }
              frame #9 {
                n214 = Not Equal To 0?(x=w409) -> (x != 0?=→"ON/OFF":bool)
              }
            }
            n215 = case shown="True" "New Button" {
              frame False {
              }
              frame True {
                n216 = property on="Waveform T" class="WFChart (strict)"("History Data"=dynamicdata[] []) -> ()  [unwired: 2 in, 2 out]
              }
            }
          }
        }
      }
      frame #2 {
        n217 = case shown="True" "Ch Max" {
          frame False {
            w428 = 1.0 ("Set ChM")
            n218 = local write "Cycles"(w428) -> ()
            n219 = local write "Set ChM"(w428) -> ()
          }
          frame True {
            n220 = local write "ISO Start"(FALSE ("ISO Start")) -> ()
            n221 = local write "V V Start"(FALSE ("V V Start")) -> ()
            n222 = local write "SP-vol-01"("Pressure Max") -> ()
            n223 = case shown="False" "Save Discharge" {
              frame False {
              }
              frame True {
              }
            }
          }
        }
        n224 = case shown="True" "V V Start" {
          frame False {
          }
          frame True {
            n225 = property on="Set v v" class="DigNum (strict)"() -> ("Value"=w440:dbl)  [unwired: 2 in, 2 out]
            n226 = local write "total Time(min)"(1.0 ("total Time(min)")) -> ()
            n227 = local write "ISO Start"(FALSE ("ISO Start")) -> ()
            n228 = local write "Ch Max"(FALSE ("Ch Max")) -> ()
            n229 = local write "t-vacuo (s)"(60.0 ("t-vacuo (s)")) -> ()
            n230 = local write "total Time(min) 2"(30.0 ("total Time(min) 2")) -> ()
            n231 = local write "Mininum Slope 2"(0.0001 ("Mininum Slope 2")) -> ()
            n232 = Divide(x="Pmax", y="Npoint") -> (x/y=w443:dbl)
            "Inter P" <- w443
            n233 = Equal?(x=w440, y=1.0) -> (x = y?=w442:bool)
            n234 = case shown="True" w442 {
              tunnel: w443 -> [w447 w449]
              tunnel: w440 -> [w448 _]
              tunnel: [w446 w449] -> w439
              frame False {
                n235 = Multiply(x=w447, y=w448) -> (x*y=w446:dbl)
                n236 = local write "SP-vol-01"(w446) -> ()
              }
              frame True {
                n237 = local write "SP-vol-01"(w449) -> ()
              }
            }
            "set P" <- w439
          }
        }
        n238 = case shown="True" "ISO Start" {
          frame False {
          }
          frame True {
            n239 = property on="Set ISO" class="DigNum (strict)"() -> ("Value"=w418:dbl)  [unwired: 2 in, 2 out]
            n240 = local write "Ch Max"(FALSE ("Ch Max")) -> ()
            n241 = local write "V V Start"(FALSE ("V V Start")) -> ()
            n242 = case shown="True" "SetP Array" {
              tunnel: w418 -> [w420 w424]
              tunnel: [w419 w427] -> w417
              frame False {
                n243 = Divide(x="Pmax 2", y="Npoint 2") -> (x/y=w421:dbl)
                "Inter P 2" <- w421
                n244 = Multiply(x=w421, y=w420) -> (x*y=w419:dbl)
              }
              frame True {
                n245 = Decrement(x=w424) -> (x-1=w425:dbl)
                n246 = Index Array(array="array", index=w425) -> (element=w427:dbl)
              }
            }
            "set P ISO" <- w417
            n247 = local write "SP-vol-01"(w417) -> ()
          }
        }
      }
      frame #3 {
        n248 = case shown="True" "PCS" {
          selector: "PCS" -> [_ w451]
          frame False {
          }
          frame True {
            n249 = flat-sequence {
              tunnel: w451 -> [w453]
              frame #0 {
                n250 = property on="Discharge" class="Bool (strict)"() -> ("Value"=w452:bool)  [unwired: 2 in, 2 out]
                n251 = case shown="False" w452 {
                  tunnel: [w455 FALSE] -> w454
                  tunnel: w453 -> [w456 _]
                  frame False {
                    n252 = Or(x=w456, y="Charge") -> (x .or. y?=w455:bool)
                    n253 = local write "Charge"(w455) -> ()
                  }
                  frame True {
                  }
                }
                n254 = case shown="False" w454 {
                  frame False {
                  }
                  frame True {
                    n255 = flat-sequence {
                      tunnel: [w470] -> w460
                      tunnel: [w465] -> w459
                      tunnel: w460 -> [w483]
                      tunnel: w459 -> [w480]
                      frame #0 {
                        n256 = call "data2byte.vi"("argument"=1.0 ("number"), "new function"=100.0) -> ("protocol"=w461:string)  [unwired: 8 in, 1 out]
                        n257 = call "Advanced Serial.vi"("Write"=TRUE ("write"), "string to write"=w461) -> ()  [unwired: 3 in, 7 out]
                      }
                      frame #1 {
                        n258 = while {
                          tunnel: [w478] -> w470
                          tunnel: [w473] -> w467
                          tunnel: [w477] -> w471
                          tunnel: [w475] -> w466
                          tunnel: [w474] -> w469
                          tunnel: [w476] -> w468
                          tunnel: [w473] -> w465
                          stop <- w479 stop-if-true
                          n259 = call "Advanced Serial.vi"() -> ("RTD-02 (ºC)"=w474:sgl, "RTD-01 (ºC)"=w475:sgl, "vacuo (mBar)"=w473:dbl, "P02 (Bar)"=w477:dbl, "RTD-chamber (ºC)"=w476:sgl, "P01 (Bar)"=w478:dbl, "32bytes"=w479:bool)  [unwired: 5 in]
                        }
                        n260 = local write "Vol01"(w470) -> ()
                        n261 = local write "Pcin"(w470) -> ()
                        n262 = local write "Vol02"(w471) -> ()
                        n263 = Merge Signals(w470, w471, w467, w466, w469, w468, w470) -> (w472:dynamicdata)
                        n264 = local write "RTD-01 (ºC)"(w466) -> ()
                        n265 = local write "RTD-02 (ºC)"(w469) -> ()
                        n266 = local write "RTD-chamber (ºC)"(w468) -> ()
                        n267 = local write "graph_completo"(w472) -> ()
                      }
                      frame #2 {
                        n268 = case shown="\"Carga Chamber\"" "command" {
                          tunnel: w483 -> [w485 w729 w996]
                          tunnel: "SP-vol-01" -> [w486 _ w999]
                          tunnel: w480 -> [_ w726 _]
                          frame "Carga vol01" {
                            n269 = Greater?(x=w486, y=w485) -> (0:w484:bool)
                            n270 = case shown="True" w484 {
                              frame False {
                                n271 = flat-sequence {
                                frame #0 {
                                n272 = call "data2byte.vi"("argument"=0.0 ("number"), "new function"=4.0) -> ("protocol"=w487:string)  [unwired: 8 in, 1 out]
                                n273 = call "Advanced Serial.vi"("Write"=TRUE ("write"), "string to write"=w487) -> ()  [unwired: 3 in, 7 out]
                                }
                                frame #1 {
                                n274 = Wait Until Next ms Multiple(millisecond multiple=u32 5) -> ()  [unwired: 1 out]
                                }
                                frame #2 {
                                n275 = while {
                                tunnel: [w563] -> w496
                                tunnel: [w562] -> w502
                                tunnel: [w561] -> w495
                                tunnel: [w560] -> w494
                                tunnel: [w559] -> w493
                                tunnel: [w558] -> w492
                                stop <- w564 stop-if-true
                                n276 = call "Advanced Serial.vi"() -> ("RTD-02 (ºC)"=w559:sgl, "RTD-01 (ºC)"=w560:sgl, "vacuo (mBar)"=w562:dbl, "P02 (Bar)"=w561:dbl, "RTD-chamber (ºC)"=w558:sgl, "P01 (Bar)"=w563:dbl, "32bytes"=w564:bool)  [unwired: 5 in]
                                }
                                n277 = property on="ISO Start" class="Bool (strict)"() -> ("Value"=w498:bool)  [unwired: 2 in, 2 out]
                                n278 = property on="Ch Max" class="Bool (strict)"() -> ("Value"=w500:bool)  [unwired: 2 in, 2 out]
                                n279 = local write "initialize"(TRUE ("initialize 2")) -> ()
                                n280 = local write "cont"(dbl[] [] ("PCv1")) -> ()
                                n281 = local write "count 2"(u32[] [] ("output array 2")) -> ()
                                n282 = local write "PCv1 completo"(dbl[] [] ("tempo carga")) -> ()
                                n283 = local write "derivada 2"(dbl[] [] ("PCv1")) -> ()
                                n284 = local write "t completo"(dbl[] [] ("PCv1")) -> ()
                                n285 = local write "SlopArray"(dbl[] [] ("PCv1")) -> ()
                                n286 = Or(x=w500, y=w498) -> (x .or. y?=w499:bool)
                                n287 = property on="Kinetic Save" class="Bool (strict)"() -> ("Value"=w497:bool)  [unwired: 2 in, 2 out]
                                n288 = local write "command"("Carga Chamber" ("String")) -> ()
                                n289 = local write "Vol01"(w496) -> ()
                                n290 = local write "Pcin"(w496) -> ()
                                n291 = local write "Vol02"(w495) -> ()
                                n292 = property on="V V Start" class="Bool (strict)"() -> ("Value"=w501:bool)  [unwired: 2 in, 2 out]
                                n293 = case shown="True" w501 {
                                tunnel: w496 -> [_ w549]
                                frame False {
                                }
                                frame True {
                                w550 = "\t"
                                n294 = property on="Set v v" class="DigNum (strict)"() -> ("Value"=w553:dbl)  [unwired: 2 in, 2 out]
                                n295 = Number To Fractional String(number=w549, precision (6)=i16 4) -> (F-format string=w551:string)  [unwired: 2 in]
                                n296 = Number To Fractional String(number=w553, precision (6)=i16 0) -> (F-format string=w555:string)  [unwired: 2 in]
                                n297 = Concatenate Strings(w555, w550, w551, w550) -> (w552:string)
                                n298 = property on="pathVV" class="Path"() -> ("Value"=w557:path)  [unwired: 2 in, 2 out]
                                n299 = call "write_file.vi"("text"=w552, "file path (use dialog)"=w557) -> ()  [unwired: 10 in]
                                }
                                }
                                n300 = case shown="True" w497 {
                                tunnel: w496 -> [_ w516]
                                tunnel: w495 -> [_ w515]
                                tunnel: w494 -> [_ w514]
                                tunnel: w493 -> [_ w513]
                                tunnel: w492 -> [_ w512]
                                frame False {
                                }
                                frame True {
                                w522 = "\t"
                                w519 = i16 4 ("precision (6)")
                                n301 = property on="Pcin" class="Slide (strict)"() -> ("Value"=w518:dbl)  [unwired: 2 in, 2 out]
                                n302 = Number To Fractional String(number=w516, precision (6)=w519) -> (F-format string=w530:string)  [unwired: 2 in]
                                n303 = Number To Fractional String(number=w515, precision (6)=w519) -> (F-format string=w529:string)  [unwired: 2 in]
                                n304 = Number To Fractional String(number=w514, precision (6)=w519) -> (F-format string=w527:string)  [unwired: 2 in]
                                n305 = Number To Fractional String(number=w512, precision (6)=w519) -> (F-format string=w526:string)  [unwired: 2 in]
                                n306 = Number To Fractional String(number=w513, precision (6)=w519) -> (F-format string=w525:string)  [unwired: 2 in]
                                n307 = Number To Fractional String(number=w518, precision (6)=w519) -> (F-format string=w520:string)  [unwired: 2 in]
                                n308 = Get Date/Time String(want seconds? (F)=TRUE) -> (date string=w533:string, time string=w531:string)  [unwired: 2 in]
                                n309 = Concatenate Strings(w533, "-" ("string"), w531, w522, w530, w522, "-" ("string"), w522, w529, w522, w527, w522, w526, w522, w525, w522, w520, "\r\n") -> (w524:string)
                                n310 = property on="path" class="Path"() -> ("Value"=w517:path)  [unwired: 2 in, 2 out]
                                n311 = call "write_file.vi"("text"=w524, "file path (use dialog)"=w517) -> ()  [unwired: 10 in]
                                }
                                }
                                n312 = case shown="True" w499 {
                                tunnel: w496 -> [_ w541]
                                tunnel: w498 -> [_ w534]
                                frame False {
                                }
                                frame True {
                                w538 = "\t"
                                n313 = case shown="True" w534 {
                                tunnel: [w547 w548] -> w540
                                frame False {
                                n314 = property on="Set ChM" class="DigNum (strict)"() -> ("Value"=w547:dbl)  [unwired: 2 in, 2 out]
                                }
                                frame True {
                                n315 = property on="Set ISO" class="DigNum (strict)"() -> ("Value"=w548:dbl)  [unwired: 2 in, 2 out]
                                }
                                }
                                n316 = property on="Cycles" class="DigNum (strict)"() -> ("Value"=w535:dbl)  [unwired: 2 in, 2 out]
                                n317 = Number To Fractional String(number=w541, precision (6)=i16 4) -> (F-format string=w542:string)  [unwired: 2 in]
                                n318 = Number To Fractional String(number=w535, precision (6)=i16 0) -> (F-format string=w536:string)  [unwired: 2 in]
                                n319 = Number To Fractional String(number=w540, precision (6)=i16 0) -> (F-format string=w545:string)  [unwired: 2 in]
                                n320 = Concatenate Strings(w536, w538, w545, w538, w542, w538) -> (w543:string)
                                n321 = property on="pathISO" class="Path"() -> ("Value"=w539:path)  [unwired: 2 in, 2 out]
                                n322 = call "write_file.vi"("text"=w543, "file path (use dialog)"=w539) -> ()  [unwired: 10 in]
                                }
                                }
                                n323 = Merge Signals(w496, w495, w502, w494, w493, w492, w496) -> (w503:dynamicdata)
                                n324 = local write "graph_completo"(w503) -> ()
                                }
                                frame #3 {
                                n325 = call "data2byte.vi"("argument"=1.0 ("number"), "new function"=1.0) -> ("protocol"=w565:string)  [unwired: 8 in, 1 out]
                                n326 = call "Advanced Serial.vi"("Write"=TRUE ("write"), "string to write"=w565) -> ()  [unwired: 3 in, 7 out]
                                }
                                frame #4 {
                                n327 = while {
                                tunnel: [w581] -> w569
                                tunnel: [w580] -> w570
                                tunnel: [w579] -> w575
                                tunnel: [w578] -> w571
                                tunnel: [w577] -> w572
                                tunnel: [w576] -> w573
                                stop <- w582 stop-if-true
                                n328 = call "Advanced Serial.vi"() -> ("RTD-02 (ºC)"=w577:sgl, "RTD-01 (ºC)"=w578:sgl, "vacuo (mBar)"=w580:dbl, "P02 (Bar)"=w579:dbl, "RTD-chamber (ºC)"=w576:sgl, "P01 (Bar)"=w581:dbl, "32bytes"=w582:bool)  [unwired: 5 in]
                                }
                                n329 = local write "Vol02"(w575) -> ()
                                n330 = local write "Vol01"(w569) -> ()
                                n331 = local write "Pcin"(w569) -> ()
                                n332 = Merge Signals(w569, w575, w570, w571, w572, w573, w569) -> (w574:dynamicdata)
                                n333 = local write "graph_completo"(w574) -> ()
                                }
                                }
                              }
                              frame True {
                                n334 = property on="ISO Start" class="Bool (strict)"() -> ("Value"=w583:bool)  [unwired: 2 in, 2 out]
                                n335 = case shown="True" w583 {
                                tunnel: [5.0 ("y") 10.0 ("y")] -> w587
                                frame False {
                                }
                                frame True {
                                }
                                }
                                n336 = Less?(x="cargas-vol1", y=1.0) -> (x < y?=→"Abrir Gas":bool)
                                n337 = Less?(x="cargas-vol1", y=w587) -> (x < y?=w588:bool)
                                n338 = case shown="False" w588 {
                                frame False {
                                n339 = while {
                                tunnel: [w709] -> w591
                                stop <- w710 stop-if-true
                                n340 = call "Advanced Serial.vi"() -> ("P01 (Bar)"=w709:dbl, "32bytes"=w710:bool)  [unwired: 5 in, 5 out]
                                }
                                n341 = local write "Abrir Gas"(TRUE ("Abrir Gas")) -> ()
                                n342 = local write "command"("abrir a garrafa" ("String")) -> ()
                                n343 = local write "Vol01"(w591) -> ()
                                n344 = local write "Pcin"(w591) -> ()
                                n345 = property on="SP-vol-01" class="DigNum (strict)"() -> ("Value"=w593:dbl)  [unwired: 2 in, 2 out]
                                n346 = Greater?(x=w591, y=w593) -> (0:w592:bool)
                                n347 = case shown="False" w592 {
                                tunnel: w591 -> [_ w630]
                                frame False {
                                n348 = call "SCC-manual.vi"() -> ("P01 (Bar)"=w597:dbl, "Gas2"=w598:bool)  [unwired: 10 out]
                                n349 = local write "Pcin"(w597) -> ()
                                n350 = property on="Kinetic Save" class="Bool (strict)"() -> ("Value"=w596:bool)  [unwired: 2 in, 2 out]
                                n351 = local write "Abrir Gas"(w598) -> ()
                                n352 = case shown="True" w596 {
                                frame False {
                                }
                                frame True {
                                w604 = "\t"
                                w601 = i16 4 ("precision (6)")
                                n353 = while {
                                tunnel: [w625] -> w615
                                tunnel: [w624] -> w613
                                tunnel: [w623] -> w611
                                tunnel: [w621] -> w609
                                tunnel: [w622] -> w607
                                stop <- w626 stop-if-true
                                n354 = call "Advanced Serial.vi"() -> ("RTD-02 (ºC)"=w622:sgl, "RTD-01 (ºC)"=w623:sgl, "P02 (Bar)"=w624:dbl, "RTD-chamber (ºC)"=w621:sgl, "P01 (Bar)"=w625:dbl, "32bytes"=w626:bool)  [unwired: 5 in, 1 out]
                                }
                                n355 = property on="Pcin" class="Slide (strict)"() -> ("Value"=w600:dbl)  [unwired: 2 in, 2 out]
                                n356 = Number To Fractional String(number=w600, precision (6)=w601) -> (F-format string=w602:string)  [unwired: 2 in]
                                n357 = Number To Fractional String(number=w615, precision (6)=w601) -> (F-format string=w617:string)  [unwired: 2 in]
                                n358 = Number To Fractional String(number=w613, precision (6)=w601) -> (F-format string=w616:string)  [unwired: 2 in]
                                n359 = Number To Fractional String(number=w611, precision (6)=w601) -> (F-format string=w612:string)  [unwired: 2 in]
                                n360 = Number To Fractional String(number=w609, precision (6)=w601) -> (F-format string=w610:string)  [unwired: 2 in]
                                n361 = Number To Fractional String(number=w607, precision (6)=w601) -> (F-format string=w608:string)  [unwired: 2 in]
                                n362 = Get Date/Time String(want seconds? (F)=TRUE) -> (date string=w620:string, time string=w618:string)  [unwired: 2 in]
                                n363 = Concatenate Strings(w620, "-" ("string"), w618, w604, w617, w604, "-" ("string"), w604, w616, w604, w612, w604, w610, w604, w608, w604, w602, "\r\n") -> (w606:string)
                                n364 = property on="path" class="Path"() -> ("Value"=w599:path)  [unwired: 2 in, 2 out]
                                n365 = call "write_file.vi"("text"=w606, "file path (use dialog)"=w599) -> ()  [unwired: 10 in]
                                }
                                }
                                }
                                frame True {
                                n366 = flat-sequence {
                                tunnel: w630 -> [w635]
                                tunnel: [w635] -> w629
                                tunnel: w629 -> [w636]
                                tunnel: [w636] -> w628
                                tunnel: w628 -> [w639]
                                tunnel: [w639] -> w627
                                tunnel: w627 -> [w679]
                                frame #0 {
                                n367 = call "data2byte.vi"("argument"=0.0 ("number"), "new function"=4.0) -> ("protocol"=w634:string)  [unwired: 8 in, 1 out]
                                n368 = call "Advanced Serial.vi"("Write"=TRUE ("write"), "string to write"=w634) -> ()  [unwired: 3 in, 7 out]
                                }
                                frame #1 {
                                n369 = Wait Until Next ms Multiple(millisecond multiple=u32 5) -> ()  [unwired: 1 out]
                                }
                                frame #2 {
                                n370 = local write "initialize"(TRUE ("initialize")) -> ()
                                n371 = local write "cont"(dbl[] [] ("PCv1")) -> ()
                                n372 = local write "PCv1 completo"(dbl[] [] ("tempo carga")) -> ()
                                n373 = local write "derivada 2"(dbl[] [] ("PCv1")) -> ()
                                n374 = local write "SlopArray"(dbl[] [] ("PCv1")) -> ()
                                n375 = local write "count 2"(u32[] [] ("output array 2")) -> ()
                                n376 = local write "t completo"(dbl[] [] ("PCv1")) -> ()
                                n377 = property on="Kinetic Save" class="Bool (strict)"() -> ("Value"=w638:bool)  [unwired: 2 in, 2 out]
                                n378 = case shown="True" w638 {
                                frame False {
                                }
                                frame True {
                                w653 = "\t"
                                w650 = i16 4 ("precision (6)")
                                n379 = while {
                                tunnel: [w674] -> w664
                                tunnel: [w673] -> w662
                                tunnel: [w672] -> w660
                                tunnel: [w670] -> w658
                                tunnel: [w671] -> w656
                                stop <- w675 stop-if-true
                                n380 = call "Advanced Serial.vi"() -> ("RTD-02 (ºC)"=w671:sgl, "RTD-01 (ºC)"=w672:sgl, "P02 (Bar)"=w673:dbl, "RTD-chamber (ºC)"=w670:sgl, "P01 (Bar)"=w674:dbl, "32bytes"=w675:bool)  [unwired: 5 in, 1 out]
                                }
                                n381 = property on="Pcin" class="Slide (strict)"() -> ("Value"=w649:dbl)  [unwired: 2 in, 2 out]
                                n382 = Number To Fractional String(number=w649, precision (6)=w650) -> (F-format string=w651:string)  [unwired: 2 in]
                                n383 = Number To Fractional String(number=w664, precision (6)=w650) -> (F-format string=w666:string)  [unwired: 2 in]
                                n384 = Number To Fractional String(number=w662, precision (6)=w650) -> (F-format string=w665:string)  [unwired: 2 in]
                                n385 = Number To Fractional String(number=w660, precision (6)=w650) -> (F-format string=w661:string)  [unwired: 2 in]
                                n386 = Number To Fractional String(number=w658, precision (6)=w650) -> (F-format string=w659:string)  [unwired: 2 in]
                                n387 = Number To Fractional String(number=w656, precision (6)=w650) -> (F-format string=w657:string)  [unwired: 2 in]
                                n388 = Get Date/Time String(want seconds? (F)=TRUE) -> (date string=w669:string, time string=w667:string)  [unwired: 2 in]
                                n389 = Concatenate Strings(w669, "-" ("string"), w667, w653, w666, w653, "-" ("string"), w653, w665, w653, w661, w653, w659, w653, w657, w653, w651, "\r\n") -> (w655:string)
                                n390 = property on="path" class="Path"() -> ("Value"=w648:path)  [unwired: 2 in, 2 out]
                                n391 = call "write_file.vi"("text"=w655, "file path (use dialog)"=w648) -> ()  [unwired: 10 in]
                                }
                                }
                                n392 = local write "command"("Carga Chamber" ("String")) -> ()
                                }
                                frame #3 {
                                n393 = property on="V V Start" class="Bool (strict)"() -> ("Value"=w680:bool)  [unwired: 2 in, 2 out]
                                n394 = property on="ISO Start" class="Bool (strict)"() -> ("Value"=w676:bool)  [unwired: 2 in, 2 out]
                                n395 = property on="Ch Max" class="Bool (strict)"() -> ("Value"=w678:bool)  [unwired: 2 in, 2 out]
                                n396 = case shown="True" w680 {
                                tunnel: w679 -> [_ w696]
                                frame False {
                                }
                                frame True {
                                w697 = "\t"
                                n397 = property on="Set v v" class="DigNum (strict)"() -> ("Value"=w700:dbl)  [unwired: 2 in, 2 out]
                                n398 = Number To Fractional String(number=w696, precision (6)=i16 4) -> (F-format string=w698:string)  [unwired: 2 in]
                                n399 = Number To Fractional String(number=w700, precision (6)=i16 0) -> (F-format string=w702:string)  [unwired: 2 in]
                                n400 = Concatenate Strings(w702, w697, w698, w697) -> (w699:string)
                                n401 = property on="pathVV" class="Path"() -> ("Value"=w704:path)  [unwired: 2 in, 2 out]
                                n402 = call "write_file.vi"("text"=w699, "file path (use dialog)"=w704) -> ()  [unwired: 10 in]
                                }
                                }
                                n403 = Or(x=w678, y=w676) -> (x .or. y?=w677:bool)
                                n404 = case shown="True" w677 {
                                tunnel: w679 -> [_ w688]
                                tunnel: w676 -> [_ w682]
                                frame False {
                                }
                                frame True {
                                w686 = "\t"
                                n405 = case shown="True" w682 {
                                tunnel: [w694 w695] -> w681
                                frame False {
                                n406 = property on="Set ChM" class="DigNum (strict)"() -> ("Value"=w694:dbl)  [unwired: 2 in, 2 out]
                                }
                                frame True {
                                n407 = property on="Set ISO" class="DigNum (strict)"() -> ("Value"=w695:dbl)  [unwired: 2 in, 2 out]
                                }
                                }
                                n408 = property on="Cycles" class="DigNum (strict)"() -> ("Value"=w683:dbl)  [unwired: 2 in, 2 out]
                                n409 = Number To Fractional String(number=w688, precision (6)=i16 4) -> (F-format string=w689:string)  [unwired: 2 in]
                                n410 = Number To Fractional String(number=w683, precision (6)=i16 0) -> (F-format string=w684:string)  [unwired: 2 in]
                                n411 = Number To Fractional String(number=w681, precision (6)=i16 0) -> (F-format string=w692:string)  [unwired: 2 in]
                                n412 = Concatenate Strings(w684, w686, w692, w686, w689, w686) -> (w690:string)
                                n413 = property on="pathISO" class="Path"() -> ("Value"=w687:path)  [unwired: 2 in, 2 out]
                                n414 = call "write_file.vi"("text"=w690, "file path (use dialog)"=w687) -> ()  [unwired: 10 in]
                                }
                                }
                                }
                                frame #4 {
                                n415 = call "data2byte.vi"("argument"=1.0 ("number"), "new function"=1.0) -> ("protocol"=w705:string)  [unwired: 8 in, 1 out]
                                n416 = call "Advanced Serial.vi"("Write"=TRUE ("write"), "string to write"=w705) -> ()  [unwired: 3 in, 7 out]
                                }
                                }
                                }
                                }
                                }
                                frame True {
                                n417 = flat-sequence {
                                tunnel: [w721] -> w711
                                tunnel: w711 -> [w724]
                                frame #0 {
                                n418 = stacked-sequence {
                                frame #0 {
                                n419 = call "data2byte.vi"("argument"=1.0 ("number"), "new function"=4.0) -> ("protocol"=w715:string)  [unwired: 8 in, 1 out]
                                n420 = call "Advanced Serial.vi"("Write"=TRUE ("write"), "string to write"=w715) -> ()  [unwired: 3 in, 7 out]
                                }
                                frame #1 {
                                n421 = Wait Until Next ms Multiple(millisecond multiple=u32 5) -> ()  [unwired: 1 out]
                                }
                                frame #2 {
                                n422 = call "data2byte.vi"("argument"=0.0 ("number"), "new function"=4.0) -> ("protocol"=w720:string)  [unwired: 8 in, 1 out]
                                n423 = call "Advanced Serial.vi"("Write"=TRUE ("write"), "string to write"=w720) -> ()  [unwired: 3 in, 7 out]
                                }
                                }
                                }
                                frame #1 {
                                n424 = property on="cargas-vol1" class="DigNum (strict)"() -> ("Value"=w722:dbl)  [unwired: 2 in, 2 out]
                                n425 = local write "command"("Carga vol01" ("String")) -> ()
                                n426 = Increment(x=w722) -> (x+1=w721:dbl)
                                }
                                frame #2 {
                                n427 = property on="cargas-vol1" class="DigNum (strict)"("Value"=w724) -> ()  [unwired: 2 in, 2 out]
                                n428 = Wait Until Next ms Multiple(millisecond multiple=u32 1000) -> ()  [unwired: 1 out]
                                }
                                }
                                }
                                }
                              }
                            }
                          }
                          frame "Carga Chamber" {
                            n429 = flat-sequence {
                              tunnel: w729 -> [w734]
                              tunnel: [w734] -> w728
                              tunnel: [w730] -> w727
                              tunnel: w726 -> [w730]
                              tunnel: w728 -> [w770]
                              tunnel: w727 -> [w750]
                              frame #0 {
                                n430 = property on="Vol01" class="Slide (strict)"() -> ("Value"=w731:dbl)  [unwired: 2 in, 2 out]
                                n431 = property on="slope" class="DigNum (strict)"() -> ("Value"=w732:dbl)  [unwired: 2 in, 2 out]
                                n432 = property on="x >= y?" class="Bool (strict)"() -> ("Value"=w733:bool)  [unwired: 2 in, 2 out]
                                n433 = local write "Pcin"(w731) -> ()
                                n434 = case shown="True" w733 {
                                tunnel: w732 -> [_ w737]
                                frame False {
                                }
                                frame True {
                                n435 = Build Array(w737) -> (w745:dbl[])
                                n436 = property on="size(s)" class="DigNum (strict)"() -> ("Value"=w740:i32)  [unwired: 2 in, 2 out]
                                n437 = local write "cargas-vol1"(0.0 ("cargas")) -> ()
                                n438 = local write "Abrir Gas"(FALSE ("Abrir Gas")) -> ()
                                n439 = local write "count"(u32[] [] ("output array 2")) -> ()
                                n440 = local write "t carga"(dbl[] [] ("tempo carga")) -> ()
                                n441 = local write "PCv1"(dbl[] [] ("PCv1")) -> ()
                                n442 = Increment(x=w740) -> (x+1=w742:i32)
                                n443 = property on="SlopArray" class="Arr (strict)"() -> ("Value"=w746:dbl[])  [unwired: 2 in, 2 out]
                                n444 = Insert Into Array(array=w746, new element=w745) -> (→"SlopArray":dbl[])  [unwired: 1 in]
                                n445 = Build Array(w742) -> (w744:i32[])
                                n446 = property on="cont" class="Arr (strict)"() -> ("Value"=w743:dbl[])  [unwired: 2 in, 2 out]
                                n447 = Insert Into Array(array=w743, new element=w744) -> (w738:dbl[])  [unwired: 1 in]
                                "cont" <- w738
                                n448 = Array Size(array=w738) -> (size(s)=→"size(s)":i32)
                                }
                                }
                                n449 = local write "Chamber"(w731) -> ()
                              }
                              frame #1 {
                                n450 = Build Array(w770) -> (w783:dbl[])
                                n451 = property on="size(s)" class="DigNum (strict)"() -> ("Value"=w772:i32)  [unwired: 2 in, 2 out]
                                n452 = Tick Count (ms)() -> (millisecond timer value=w776:u32)
                                n453 = Tick Count (ms)() -> (millisecond timer value=w802:u32)
                                n454 = property on="t completo" class="Arr (strict)"() -> ("Value"=w785:dbl[])  [unwired: 2 in, 2 out]
                                n455 = property on="Kinetic Save" class="Bool (strict)"() -> ("Value"=w751:bool)  [unwired: 2 in, 2 out]
                                n456 = property on="PCv1 completo" class="Arr (strict)"() -> ("Value"=w784:dbl[])  [unwired: 2 in, 2 out]
                                n457 = Build Array(w776) -> (w775:u32[])
                                n458 = property on="PCv1" class="Arr (strict)"() -> ("Value"=w804:dbl[])  [unwired: 2 in, 2 out]
                                n459 = Build Array(w802) -> (w787:u32[])
                                n460 = Multiply(x=w772, y=10 ("t(s)")) -> (x*y=w771:i32)
                                n461 = case shown="True" w751 {
                                frame False {
                                }
                                frame True {
                                w810 = "\t"
                                w807 = i16 4 ("precision (6)")
                                n462 = while {
                                tunnel: [w831] -> w821
                                tunnel: [w830] -> w819
                                tunnel: [w829] -> w817
                                tunnel: [w827] -> w815
                                tunnel: [w828] -> w813
                                stop <- w832 stop-if-true
                                n463 = call "Advanced Serial.vi"() -> ("RTD-02 (ºC)"=w828:sgl, "RTD-01 (ºC)"=w829:sgl, "P02 (Bar)"=w830:dbl, "RTD-chamber (ºC)"=w827:sgl, "P01 (Bar)"=w831:dbl, "32bytes"=w832:bool)  [unwired: 5 in, 1 out]
                                }
                                n464 = property on="Pcin" class="Slide (strict)"() -> ("Value"=w805:dbl)  [unwired: 2 in, 2 out]
                                n465 = Number To Fractional String(number=w805, precision (6)=w807) -> (F-format string=w808:string)  [unwired: 2 in]
                                n466 = Number To Fractional String(number=w821, precision (6)=w807) -> (F-format string=w823:string)  [unwired: 2 in]
                                n467 = Number To Fractional String(number=w819, precision (6)=w807) -> (F-format string=w822:string)  [unwired: 2 in]
                                n468 = Number To Fractional String(number=w817, precision (6)=w807) -> (F-format string=w818:string)  [unwired: 2 in]
                                n469 = Number To Fractional String(number=w815, precision (6)=w807) -> (F-format string=w816:string)  [unwired: 2 in]
                                n470 = Number To Fractional String(number=w813, precision (6)=w807) -> (F-format string=w814:string)  [unwired: 2 in]
                                n471 = Get Date/Time String(want seconds? (F)=TRUE) -> (date string=w826:string, time string=w824:string)  [unwired: 2 in]
                                n472 = Concatenate Strings(w826, "-" ("string"), w824, w810, w823, w810, "-" ("string"), w810, w822, w810, w818, w810, w816, w810, w814, w810, w808, "\r\n") -> (w812:string)
                                n473 = property on="path" class="Path"() -> ("Value"=w806:path)  [unwired: 2 in, 2 out]
                                n474 = call "write_file.vi"("text"=w812, "file path (use dialog)"=w806) -> ()  [unwired: 10 in]
                                }
                                }
                                n475 = Insert Into Array(array=w784, new element=w783) -> (w777:dbl[])  [unwired: 1 in]
                                "PCv1 completo" <- w777
                                n476 = Insert Into Array(array=w804, new element=w783) -> (w756:dbl[])  [unwired: 1 in]
                                "PCv1" <- w756
                                n477 = property on="count" class="Arr (strict)"() -> ("Value"=w803:u32[])  [unwired: 2 in, 2 out]
                                n478 = property on="count 2" class="Arr (strict)"() -> ("Value"=w788:u32[])  [unwired: 2 in, 2 out]
                                n479 = Insert Into Array(array=w788, new element=w775) -> (w793:u32[])  [unwired: 1 in]
                                "count 2" <- w793
                                n480 = Insert Into Array(array=w803, new element=w787) -> (w795:u32[])  [unwired: 1 in]
                                "count" <- w795
                                n481 = Array Max & Min(array=w793) -> (max value=w789:u32, min value=w790:u32)  [unwired: 2 out]
                                n482 = Array Max & Min(array=w795) -> (max value=w801:u32, min value=w800:u32)  [unwired: 2 out]
                                n483 = Subtract(x=w789, y=w790) -> (x-y=w792:u32)
                                n484 = Subtract(x=w801, y=w800) -> (x-y=w798:u32)
                                n485 = Divide(x=w798, y=1000.0) -> (x/y=w794:dbl)
                                n486 = Divide(x=w792, y=60000.0) -> (x/y=w764:dbl)
                                "time (min)" <- w764
                                n487 = Greater Or Equal?(x=w794, y=w771) -> (x >= y?=w760:bool)
                                "x >= y?" <- w760
                                n488 = Build Array(w794) -> (w796:dbl[])
                                n489 = call <vilib>:"Derivative x(t) PtByPt.vi"("initialize"="initialize", "dt"=w764, "x"=w770) -> ("dx/dt"=w763:dbl)  [unwired: 1 in, 1 out]
                                "dp/dt" <- w763
                                n490 = Build Array(w764) -> (w786:dbl[])
                                n491 = property on="t carga" class="Arr (strict)"() -> ("Value"=w797:dbl[])  [unwired: 2 in, 2 out]
                                n492 = Insert Into Array(array=w797, new element=w796) -> (w757:dbl[])  [unwired: 1 in]
                                "t carga" <- w757
                                n493 = Insert Into Array(array=w785, new element=w786) -> (w767:dbl[])  [unwired: 1 in]
                                "t completo" <- w767
                                n494 = Bundle("Value"=w767, "Value"=w777) -> (w782:cluster{"Value":dbl[], "Value":dbl[]})  [unwired: 1 in]
                                n495 = Build Array(w763) -> (w769:dbl[])
                                n496 = Bundle("Value"=w757, "Value"=w756) -> (w781:cluster{"Value":dbl[], "Value":dbl[]})  [unwired: 1 in]
                                n497 = call <vilib>:"General Polynomial Fit.vi"("Y"=w756, "polynomial order"=0, "X"=w757) -> ("Best Polynomial Fit"=w754:dbl[], "Polynomial Coefficients"=w753:dbl[])  [unwired: 9 in, 2 out]
                                n498 = call <vilib>:"Linear Fit.vi"("Y"=w756, "X"=w757) -> ("Best Linear Fit"=w774:dbl[], "slope"=w761:dbl)  [unwired: 9 in, 3 out]
                                "slope" <- w761
                                n499 = property on="derivada 2" class="Arr (strict)"() -> ("Value"=w768:dbl[])  [unwired: 2 in, 2 out]
                                n500 = Insert Into Array(array=w768, new element=w769) -> (w766:dbl[])  [unwired: 1 in]
                                "derivada 2" <- w766
                                n501 = Bundle("Value"=w757, "Best Polynomial Fit"=w754) -> (w758:T8)  [unwired: 1 in]
                                n502 = Index Array(array=w753) -> (element=w752:dbl)  [unwired: 1 in]
                                n503 = local write "Pfit"(w752) -> ()
                                n504 = Bundle("Value"=w757, "Best Linear Fit"=w774) -> (w780:cluster{"Value":dbl[], "Best Linear Fit":dbl[]})  [unwired: 1 in]
                                n505 = case shown="True" w760 {
                                tunnel: w764 -> [_ w845]
                                tunnel: w763 -> [_ w843]
                                tunnel: "dp/dt min" -> [_ w842]
                                tunnel: w761 -> [_ w836]
                                tunnel: w752 -> [_ w834]
                                tunnel: w750 -> [_ w833]
                                frame False {
                                }
                                frame True {
                                n506 = Less Or Equal?(x=w843, y=w842) -> (x <= y?=w840:bool)
                                n507 = Absolute Value(x=w836) -> (abs(x)=w837:dbl)
                                n508 = Greater Or Equal?(x=w845, y="total Time(min)") -> (x >= y?=w846:bool)
                                n509 = Less Or Equal?(x=w837, y="Mininum Slope") -> (x <= y?=w839:bool)
                                n510 = Or(x=w840, y=w839) -> (x .or. y?=w841:bool)
                                n511 = Or(x=w846, y=w841) -> (x .or. y?=w835:bool)
                                n512 = case shown="True" w835 {
                                tunnel: w835 -> [_ w862]
                                tunnel: w834 -> [_ w858]
                                tunnel: w833 -> [_ w847]
                                frame False {
                                }
                                frame True {
                                n513 = flat-sequence {
                                tunnel: w862 -> [_]
                                tunnel: [w867] -> w859
                                tunnel: w858 -> [w867]
                                tunnel: [w872] -> w860
                                tunnel: w859 -> [w871]
                                tunnel: [w871] -> w856
                                tunnel: [w870] -> w855
                                tunnel: [w869] -> w854
                                tunnel: [w868] -> w853
                                tunnel: [w891] -> w857
                                tunnel: w860 -> [w891]
                                tunnel: w856 -> [w886]
                                tunnel: w855 -> [w885]
                                tunnel: w854 -> [w887]
                                tunnel: w853 -> [w888]
                                tunnel: [w890] -> w850
                                tunnel: [w884] -> w849
                                tunnel: [w934] -> w861
                                tunnel: w857 -> [w934]
                                tunnel: [w933] -> w851
                                tunnel: w850 -> [w933]
                                tunnel: w849 -> [w932]
                                tunnel: [w932] -> w848
                                tunnel: w861 -> [w939]
                                tunnel: [w938] -> w852
                                tunnel: w851 -> [w938]
                                tunnel: w848 -> [w937]
                                tunnel: w847 -> [w936]
                                tunnel: w852 -> [w982]
                                frame #0 {
                                n514 = call "data2byte.vi"("argument"=0.0 ("number"), "new function"=1.0) -> ("protocol"=w863:string)  [unwired: 8 in, 1 out]
                                n515 = call "Advanced Serial.vi"("Write"=TRUE ("write"), "string to write"=w863) -> ()  [unwired: 3 in, 7 out]
                                }
                                frame #1 {
                                n516 = property on="RTD-01 (ºC)" class="DigNum (strict)"() -> ("Value"=w870:sgl)  [unwired: 2 in, 2 out]
                                n517 = property on="RTD-02 (ºC)" class="DigNum (strict)"() -> ("Value"=w868:sgl)  [unwired: 2 in, 2 out]
                                n518 = property on="V V Start" class="Bool (strict)"() -> ("Value"=w872:bool)  [unwired: 2 in, 2 out]
                                n519 = property on="RTD-chamber (ºC)" class="DigNum (strict)"() -> ("Value"=w869:sgl)  [unwired: 2 in, 2 out]
                                n520 = case shown="True" w872 {
                                tunnel: w871 -> [_ w875]
                                tunnel: w870 -> [_ w874]
                                tunnel: w869 -> [_ w873]
                                frame False {
                                }
                                frame True {
                                w880 = "\t"
                                w881 = i16 4 ("precision (6)")
                                n521 = Number To Fractional String(number=w875, precision (6)=w881) -> (F-format string=w877:string)  [unwired: 2 in]
                                n522 = Number To Fractional String(number=w874, precision (6)=w881) -> (F-format string=w879:string)  [unwired: 2 in]
                                n523 = Number To Fractional String(number=w873, precision (6)=w881) -> (F-format string=w882:string)  [unwired: 2 in]
                                n524 = Concatenate Strings(w877, w880, w879, w880, w882, "\r\n") -> (w878:string)
                                n525 = property on="pathVV" class="Path"() -> ("Value"=w876:path)  [unwired: 2 in, 2 out]
                                n526 = call "write_file.vi"("text"=w878, "file path (use dialog)"=w876) -> ()  [unwired: 10 in]
                                }
                                }
                                }
                                frame #2 {
                                n527 = property on="ISO Start" class="Bool (strict)"() -> ("Value"=w884:bool)  [unwired: 2 in, 2 out]
                                n528 = local write "command"("StartDesc" ("String")) -> ()
                                n529 = case shown="True" w884 {
                                tunnel: w886 -> [_ w904]
                                tunnel: w885 -> [_ w903]
                                tunnel: w887 -> [_ w902]
                                tunnel: w888 -> [_ w894]
                                frame False {
                                }
                                frame True {
                                w897 = "\t"
                                w895 = i16 4 ("precision (6)")
                                n530 = Number To Fractional String(number=w904, precision (6)=w895) -> (F-format string=w905:string)  [unwired: 2 in]
                                n531 = Number To Fractional String(number=w903, precision (6)=w895) -> (F-format string=w900:string)  [unwired: 2 in]
                                n532 = Number To Fractional String(number=w902, precision (6)=w895) -> (F-format string=w898:string)  [unwired: 2 in]
                                n533 = Number To Fractional String(number=w894, precision (6)=w895) -> (F-format string=w893:string)  [unwired: 2 in]
                                n534 = Concatenate Strings(w905, w897, "==>" ("string"), w897, w900, w897, w898, w897, w893, "\r\n") -> (w906:string)
                                n535 = property on="pathISO" class="Path"() -> ("Value"=w901:path)  [unwired: 2 in, 2 out]
                                n536 = call "write_file.vi"("text"=w906, "file path (use dialog)"=w901) -> ()  [unwired: 10 in]
                                }
                                }
                                n537 = property on="Save Discharge" class="Bool (strict)"() -> ("Value"=w889:bool)  [unwired: 2 in, 2 out]
                                n538 = property on="Ch Max" class="Bool (strict)"() -> ("Value"=w890:bool)  [unwired: 2 in, 2 out]
                                n539 = case shown="True" w890 {
                                tunnel: w886 -> [_ w911]
                                tunnel: w885 -> [_ w910]
                                tunnel: w887 -> [_ w909]
                                tunnel: w888 -> [_ w908]
                                tunnel: w889 -> [_ w907]
                                frame False {
                                }
                                frame True {
                                n540 = case shown="False" w907 {
                                tunnel: w911 -> [w923 w928]
                                tunnel: w910 -> [w922 _]
                                tunnel: w909 -> [w921 _]
                                tunnel: w908 -> [w913 _]
                                frame False {
                                w916 = "\t"
                                w914 = i16 4 ("precision (6)")
                                n541 = Number To Fractional String(number=w923, precision (6)=w914) -> (F-format string=w924:string)  [unwired: 2 in]
                                n542 = Number To Fractional String(number=w922, precision (6)=w914) -> (F-format string=w919:string)  [unwired: 2 in]
                                n543 = Number To Fractional String(number=w921, precision (6)=w914) -> (F-format string=w917:string)  [unwired: 2 in]
                                n544 = Number To Fractional String(number=w913, precision (6)=w914) -> (F-format string=w912:string)  [unwired: 2 in]
                                n545 = Concatenate Strings(w924, w916, "==>" ("string"), w916, w919, w916, w917, w916, w912, "\r\n") -> (w925:string)
                                n546 = property on="pathISO" class="Path"() -> ("Value"=w920:path)  [unwired: 2 in, 2 out]
                                n547 = call "write_file.vi"("text"=w925, "file path (use dialog)"=w920) -> ()  [unwired: 10 in]
                                }
                                frame True {
                                n548 = Number To Fractional String(number=w928, precision (6)=i16 4) -> (F-format string=w929:string)  [unwired: 2 in]
                                n549 = Concatenate Strings(w929, "\t") -> (w931:string)
                                n550 = property on="pathISO" class="Path"() -> ("Value"=w930:path)  [unwired: 2 in, 2 out]
                                n551 = call "write_file.vi"("text"=w931, "file path (use dialog)"=w930) -> ()  [unwired: 10 in]
                                }
                                }
                                }
                                }
                                }
                                frame #3 {
                                n552 = Wait Until Next ms Multiple(millisecond multiple=u32 5) -> ()  [unwired: 1 out]
                                }
                                frame #4 {
                                n553 = case shown="True" w939 {
                                selector: w939 -> [w971 w972]
                                frame False {
                                n554 = local write "Charge"(w971) -> ()
                                }
                                frame True {
                                n555 = local write "Charge"(w972) -> ()
                                n556 = property on="Npoint" class="DigNum (strict)"() -> ("Value"=w975:i32)  [unwired: 2 in, 2 out]
                                n557 = property on="Set v v" class="DigNum (strict)"() -> ("Value"=w973:dbl)  [unwired: 2 in, 2 out]
                                n558 = Greater Or Equal?(x=w973, y=w975) -> (x >= y?=w974:bool)
                                n559 = case shown="True" w974 {
                                selector: w974 -> [w976 w981]
                                tunnel: w973 -> [w977 _]
                                frame False {
                                n560 = Increment(x=w977) -> (x+1=w978:dbl)
                                n561 = local write "Discharge"(w976) -> ()
                                n562 = local write "Set v v"(w978) -> ()
                                }
                                frame True {
                                n563 = Not(x=w981) -> (.not. x?=w979:bool)
                                n564 = local write "Discharge"(w981) -> ()
                                n565 = local write "Set v v"(1.0 ("Set v v")) -> ()
                                n566 = local write "Charge"(w979) -> ()
                                n567 = local write "V V Start"(w979) -> ()
                                }
                                }
                                }
                                }
                                n568 = case shown="True" w937 {
                                selector: w937 -> [w940 w945]
                                tunnel: w936 -> [_ w941]
                                frame False {
                                n569 = local write "Charge"(w940) -> ()
                                }
                                frame True {
                                n570 = local write "Charge"(w945) -> ()
                                n571 = property on="Pmax 2" class="DigNum (strict)"() -> ("Value"=w942:i32)  [unwired: 2 in, 2 out]
                                n572 = property on="Chamber" class="Slide (strict)"() -> ("Value"=w943:dbl)  [unwired: 2 in, 2 out]
                                n573 = Greater Or Equal?(x=w943, y=w942) -> (x >= y?=w946:bool)
                                n574 = property on="Set ISO" class="DigNum (strict)"() -> ("Value"=w944:dbl)  [unwired: 2 in, 2 out]
                                n575 = case shown="True" w946 {
                                selector: w946 -> [w948 w955]
                                tunnel: w944 -> [w949 w952]
                                tunnel: w941 -> [_ w950]
                                frame False {
                                n576 = local write "Discharge"(w948) -> ()
                                n577 = Increment(x=w949) -> (x+1=w947:dbl)
                                n578 = local write "Set ISO"(w947) -> ()
                                }
                                frame True {
                                n579 = local write "Discharge"(w955) -> ()
                                n580 = flat-sequence {
                                tunnel: [w958] -> w953
                                tunnel: w952 -> [w957]
                                tunnel: [w956] -> w951
                                tunnel: w950 -> [w956]
                                tunnel: w953 -> [w960]
                                tunnel: w951 -> [w959]
                                frame #0 {
                                n581 = Increment(x=w957) -> (x+1=w958:dbl)
                                n582 = local write "Set ISO"(w958) -> ()
                                }
                                frame #1 {
                                w967 = i16 0 ("precision (6)")
                                w961 = "\t"
                                n583 = property on="Cycles" class="DigNum (strict)"() -> ("Value"=w966:dbl)  [unwired: 2 in, 2 out]
                                n584 = Number To Fractional String(number=w959, precision (6)=i16 4) -> (F-format string=w962:string)  [unwired: 2 in]
                                n585 = Number To Fractional String(number=w966, precision (6)=w967) -> (F-format string=w965:string)  [unwired: 2 in]
                                n586 = Number To Fractional String(number=w960, precision (6)=w967) -> (F-format string=w964:string)  [unwired: 2 in]
                                n587 = Concatenate Strings(w965, w961, w964, w961, "==>", w961, w962, w961) -> (w970:string)
                                n588 = property on="pathISO" class="Path"() -> ("Value"=w969:path)  [unwired: 2 in, 2 out]
                                n589 = call "write_file.vi"("text"=w970, "file path (use dialog)"=w969) -> ()  [unwired: 10 in]
                                }
                                }
                                n590 = Not(x=w955) -> (.not. x?=w954:bool)
                                n591 = local write "Charge"(w954) -> ()
                                }
                                }
                                }
                                }
                                }
                                frame #5 {
                                n592 = case shown="True" w982 {
                                selector: w982 -> [_ w984]
                                frame False {
                                }
                                frame True {
                                n593 = Not(x=w984) -> (.not. x?=w985:bool)
                                n594 = local write "Discharge"(w984) -> ()
                                n595 = local write "Charge"(w985) -> ()
                                n596 = property on="Save Discharge" class="Bool (strict)"() -> ("Value"=w983:bool)  [unwired: 2 in, 2 out]
                                n597 = case shown="False" w983 {
                                frame False {
                                n598 = property on="N cycles" class="DigNum (strict)"() -> ("Value"=w988:dbl)  [unwired: 2 in, 2 out]
                                n599 = property on="Set ChM" class="DigNum (strict)"() -> ("Value"=w991:dbl)  [unwired: 2 in, 2 out]
                                n600 = Increment(x=w991) -> (x+1=w989:dbl)
                                n601 = Add(x=w988, y=2.0 ("Cycles")) -> (x+y=w987:dbl)
                                n602 = local write "Cycles"(w989) -> ()
                                n603 = Greater?(x=w987, y=w989) -> (0:w990:bool)
                                n604 = local write "Set ChM"(w989) -> ()
                                n605 = case shown="False" w990 {
                                selector: w990 -> [w992 w994]
                                frame False {
                                w993 = 1.0 ("Cycles")
                                n606 = local write "Discharge"(w992) -> ()
                                n607 = local write "clear sample"(w992) -> ()
                                n608 = local write "Kinetic Save"(w992) -> ()
                                n609 = local write "Ch Max"(w992) -> ()
                                n610 = local write "Cycles"(w993) -> ()
                                n611 = local write "Set ChM"(w993) -> ()
                                }
                                frame True {
                                n612 = local write "Ch Max"(w994) -> ()
                                }
                                }
                                }
                                frame True {
                                w995 = FALSE ("descarga 2")
                                n613 = local write "estado"(w995) -> ()
                                n614 = local write "slop"(w995) -> ()
                                n615 = local write "descarga 2"(w995) -> ()
                                }
                                }
                                }
                                }
                                }
                                }
                                }
                                }
                                }
                                }
                                n616 = Build Array(w781, w780, w758) -> (w779:T3)
                                n617 = Bundle("Value"=w767, "Value"=w766) -> (w759:cluster{"Value":dbl[], "Value":dbl[]})  [unwired: 1 in]
                                n618 = local write "slop01"(w779) -> ()
                                n619 = Build Array(w782, w759) -> (w778:cluster{"Value":dbl[], "Value":dbl[]}[])
                                n620 = local write "fit-all"(w778) -> ()
                              }
                            }
                          }
                          frame "Start", Default {
                            n621 = Greater?(x=w999, y=w996) -> (0:w1000:bool)
                            n622 = flat-sequence {
                              tunnel: w1000 -> [w1005]
                              tunnel: [w1005] -> w998
                              tunnel: [w1003] -> w997
                              tunnel: w996 -> [w1003]
                              tunnel: w998 -> [w1027]
                              tunnel: w997 -> [w1026]
                              frame #0 {
                                n623 = local write "Abrir Gas"(FALSE ("Abrir Gas")) -> ()
                                n624 = stacked-sequence {
                                tunnel: 0.0 ("number") -> [w1007 w1011 w1014 w1018 w1022]
                                tunnel: TRUE ("write") -> [w1006 w1010 w1015 w1019 w1023]
                                frame #0 {
                                n625 = call "data2byte.vi"("argument"=w1007, "new function"=1.0) -> ("protocol"=w1008:string)  [unwired: 8 in, 1 out]
                                n626 = call "Advanced Serial.vi"("Write"=w1006, "string to write"=w1008) -> ()  [unwired: 3 in, 7 out]
                                }
                                frame #1 {
                                n627 = call "data2byte.vi"("argument"=w1011, "new function"=2.0) -> ("protocol"=w1012:string)  [unwired: 8 in, 1 out]
                                n628 = call "Advanced Serial.vi"("Write"=w1010, "string to write"=w1012) -> ()  [unwired: 3 in, 7 out]
                                }
                                frame #2 {
                                n629 = call "data2byte.vi"("argument"=w1014, "new function"=3.0) -> ("protocol"=w1016:string)  [unwired: 8 in, 1 out]
                                n630 = call "Advanced Serial.vi"("Write"=w1015, "string to write"=w1016) -> ()  [unwired: 3 in, 7 out]
                                }
                                frame #3 {
                                n631 = call "data2byte.vi"("argument"=w1018, "new function"=4.0) -> ("protocol"=w1020:string)  [unwired: 8 in, 1 out]
                                n632 = call "Advanced Serial.vi"("Write"=w1019, "string to write"=w1020) -> ()  [unwired: 3 in, 7 out]
                                }
                                frame #4 {
                                n633 = call "data2byte.vi"("argument"=w1022, "new function"=5.0) -> ("protocol"=w1024:string)  [unwired: 8 in, 1 out]
                                n634 = call "Advanced Serial.vi"("Write"=w1023, "string to write"=w1024) -> ()  [unwired: 3 in, 7 out]
                                }
                                }
                              }
                              frame #1 {
                                n635 = case shown="True" w1027 {
                                tunnel: w1026 -> [w1028 _]
                                frame False {
                                n636 = flat-sequence {
                                tunnel: [w1036] -> w1029
                                tunnel: w1028 -> [w1036]
                                tunnel: [w1037] -> w1030
                                tunnel: w1029 -> [w1037]
                                tunnel: [w1039] -> w1031
                                tunnel: w1030 -> [w1039]
                                tunnel: w1031 -> [w1051]
                                frame #0 {
                                n637 = call "data2byte.vi"("argument"=0.0 ("number"), "new function"=4.0) -> ("protocol"=w1032:string)  [unwired: 8 in, 1 out]
                                n638 = call "Advanced Serial.vi"("Write"=TRUE ("write"), "string to write"=w1032) -> ()  [unwired: 3 in, 7 out]
                                }
                                frame #1 {
                                n639 = Wait Until Next ms Multiple(millisecond multiple=u32 5) -> ()  [unwired: 1 out]
                                }
                                frame #2 {
                                n640 = local write "initialize"(TRUE ("initialize")) -> ()
                                n641 = local write "derivada 2"(dbl[] [] ("PCv1")) -> ()
                                n642 = local write "cont"(dbl[] [] ("PCv1")) -> ()
                                n643 = local write "count 2"(u32[] [] ("output array 2")) -> ()
                                n644 = local write "PCv1 completo"(dbl[] [] ("tempo carga")) -> ()
                                n645 = local write "SlopArray"(dbl[] [] ("PCv1")) -> ()
                                n646 = local write "t completo"(dbl[] [] ("PCv1")) -> ()
                                n647 = local write "command"("Carga Chamber" ("String")) -> ()
                                }
                                frame #3 {
                                n648 = property on="Ch Max" class="Bool (strict)"() -> ("Value"=w1049:bool)  [unwired: 2 in, 2 out]
                                n649 = property on="ISO Start" class="Bool (strict)"() -> ("Value"=w1048:bool)  [unwired: 2 in, 2 out]
                                n650 = property on="V V Start" class="Bool (strict)"() -> ("Value"=w1052:bool)  [unwired: 2 in, 2 out]
                                n651 = case shown="True" w1052 {
                                tunnel: w1051 -> [_ w1065]
                                frame False {
                                }
                                frame True {
                                w1066 = "\t"
                                n652 = property on="Set v v" class="DigNum (strict)"() -> ("Value"=w1069:dbl)  [unwired: 2 in, 2 out]
                                n653 = Number To Fractional String(number=w1065, precision (6)=i16 4) -> (F-format string=w1067:string)  [unwired: 2 in]
                                n654 = Number To Fractional String(number=w1069, precision (6)=i16 0) -> (F-format string=w1071:string)  [unwired: 2 in]
                                n655 = Concatenate Strings(w1071, w1066, w1067, w1066) -> (w1068:string)
                                n656 = property on="pathVV" class="Path"() -> ("Value"=w1073:path)  [unwired: 2 in, 2 out]
                                n657 = call "write_file.vi"("text"=w1068, "file path (use dialog)"=w1073) -> ()  [unwired: 10 in]
                                }
                                }
                                n658 = Or(x=w1049, y=w1048) -> (x .or. y?=w1050:bool)
                                n659 = case shown="True" w1050 {
                                tunnel: w1051 -> [_ w1059]
                                frame False {
                                }
                                frame True {
                                w1056 = "\t"
                                n660 = property on="Cycles" class="DigNum (strict)"() -> ("Value"=w1054:dbl)  [unwired: 2 in, 2 out]
                                n661 = property on="Set ChM" class="DigNum (strict)"() -> ("Value"=w1058:dbl)  [unwired: 2 in, 2 out]
                                n662 = Number To Fractional String(number=w1059, precision (6)=i16 4) -> (F-format string=w1060:string)  [unwired: 2 in]
                                n663 = Number To Fractional String(number=w1054, precision (6)=i16 0) -> (F-format string=w1055:string)  [unwired: 2 in]
                                n664 = Number To Fractional String(number=w1058, precision (6)=i16 0) -> (F-format string=w1063:string)  [unwired: 2 in]
                                n665 = Concatenate Strings(w1055, w1056, w1063, w1056, w1060, w1056) -> (w1061:string)
                                n666 = property on="pathISO" class="Path"() -> ("Value"=w1057:path)  [unwired: 2 in, 2 out]
                                n667 = call "write_file.vi"("text"=w1061, "file path (use dialog)"=w1057) -> ()  [unwired: 10 in]
                                }
                                }
                                }
                                frame #4 {
                                n668 = call "data2byte.vi"("argument"=1.0 ("number"), "new function"=1.0) -> ("protocol"=w1074:string)  [unwired: 8 in, 1 out]
                                n669 = call "Advanced Serial.vi"("Write"=TRUE ("write"), "string to write"=w1074) -> ()  [unwired: 3 in, 7 out]
                                }
                                }
                                }
                                frame True {
                                n670 = flat-sequence {
                                frame #0 {
                                n671 = local write "command"("Carga vol01" ("String")) -> ()
                                }
                                frame #1 {
                                n672 = Wait Until Next ms Multiple(millisecond multiple=u32 5) -> ()  [unwired: 1 out]
                                }
                                }
                                }
                                }
                              }
                            }
                          }
                        }
                      }
                    }
                  }
                }
              }
              frame #1 {
                n673 = case shown="True" "Discharge" {
                  frame False {
                  }
                  frame True {
                    n674 = flat-sequence {
                      tunnel: [w1090] -> w1084
                      tunnel: [w1092] -> w1083
                      tunnel: w1084 -> [w1113]
                      tunnel: w1083 -> [w1120]
                      tunnel: [w1113] -> w1082
                      tunnel: [w1112] -> w1081
                      tunnel: w1082 -> [w1136]
                      tunnel: w1081 -> [w1137]
                      frame #0 {
                        n675 = call "data2byte.vi"("argument"=1.0 ("number"), "new function"=100.0) -> ("protocol"=w1085:string)  [unwired: 8 in, 1 out]
                        n676 = call "Advanced Serial.vi"("Write"=TRUE ("write"), "string to write"=w1085) -> ()  [unwired: 3 in, 7 out]
                      }
                      frame #1 {
                        n677 = Wait Until Next ms Multiple(millisecond multiple=u32 5) -> ()  [unwired: 1 out]
                      }
                      frame #2 {
                        n678 = while {
                          tunnel: [w1109] -> w1099
                          tunnel: [w1108] -> w1092
                          tunnel: [w1104] -> w1098
                          tunnel: [w1107] -> w1097
                          tunnel: [w1106] -> w1096
                          tunnel: [w1105] -> w1095
                          tunnel: [w1104] -> w1090
                          stop <- w1110 stop-if-true
                          n679 = call "Advanced Serial.vi"() -> ("RTD-02 (ºC)"=w1106:sgl, "RTD-01 (ºC)"=w1107:sgl, "vacuo (mBar)"=w1108:dbl, "P02 (Bar)"=w1104:dbl, "RTD-chamber (ºC)"=w1105:sgl, "P01 (Bar)"=w1109:dbl, "32bytes"=w1110:bool)  [unwired: 5 in]
                        }
                        "vacuo (mBar)" <- w1092
                        n680 = local write "Vol01"(w1099) -> ()
                        n681 = local write "Vol02"(w1090) -> ()
                        n682 = property on="descarga 2" class="Bool (strict)"() -> ("Value"=w1093:bool)  [unwired: 2 in, 2 out]
                        n683 = case shown="True" w1093 {
                          tunnel: w1092 -> [w1100 _]
                          tunnel: [w1101 w1103] -> w1091
                          tunnel: w1090 -> [_ w1103]
                          frame False {
                            n684 = Multiply(x=w1100, y=0.001) -> (x*y=w1101:dbl)
                            n685 = local write "Pcin"(w1101) -> ()
                          }
                          frame True {
                            n686 = local write "Pcin"(w1103) -> ()
                          }
                        }
                        n687 = Merge Signals(w1099, w1098, w1092, w1097, w1096, w1095, w1091) -> (w1094:dynamicdata)
                        n688 = local write "graph_completo"(w1094) -> ()
                      }
                      frame #3 {
                        n689 = Less?(x=w1120, y=3.0) -> (x < y?=w1117:bool)
                        n690 = Less?(x=w1113, y=1.2) -> (x < y?=w1118:bool)
                        n691 = And(x=w1118, y=w1117) -> (x .and. y?=w1116:bool)
                        n692 = stacked-sequence {
                          tunnel: 0.0 ("number") -> [w1125 _ w1128 w1132 _]
                          tunnel: TRUE ("write") -> [w1124 _ w1129 w1133 _]
                          frame #0 {
                            n693 = call "data2byte.vi"("argument"=w1125, "new function"=1.0) -> ("protocol"=w1126:string)  [unwired: 8 in, 1 out]
                            n694 = call "Advanced Serial.vi"("Write"=w1124, "string to write"=w1126) -> ()  [unwired: 3 in, 7 out]
                          }
                          frame #1 {
                          }
                          frame #2 {
                            n695 = call "data2byte.vi"("argument"=w1128, "new function"=3.0) -> ("protocol"=w1130:string)  [unwired: 8 in, 1 out]
                            n696 = call "Advanced Serial.vi"("Write"=w1129, "string to write"=w1130) -> ()  [unwired: 3 in, 7 out]
                          }
                          frame #3 {
                            n697 = call "data2byte.vi"("argument"=w1132, "new function"=4.0) -> ("protocol"=w1134:string)  [unwired: 8 in, 1 out]
                            n698 = call "Advanced Serial.vi"("Write"=w1133, "string to write"=w1134) -> ()  [unwired: 3 in, 7 out]
                          }
                          frame #4 {
                          }
                        }
                        n699 = property on="descarga 2" class="Bool (strict)"() -> ("Value"=w1111:bool)  [unwired: 2 in, 2 out]
                        n700 = case shown="True" w1111 {
                          tunnel: w1116 -> [w1122 _]
                          tunnel: [w1122 TRUE] -> w1112
                          frame False {
                            "estado" <- w1122
                          }
                          frame True {
                          }
                        }
                      }
                      frame #4 {
                        n701 = case shown="True" w1137 {
                          tunnel: w1136 -> [w1139 w1189]
                          frame False {
                            n702 = Greater?(x=w1139, y=1.5) -> (0:w1140:bool)
                            n703 = flat-sequence {
                              tunnel: w1140 -> [w1141]
                              frame #0 {
                                n704 = case shown="True" w1141 {
                                frame False {
                                }
                                frame True {
                                n705 = flat-sequence {
                                frame #0 {
                                n706 = call "data2byte.vi"("argument"=1.0 ("number"), "new function"=5.0) -> ("protocol"=w1142:string)  [unwired: 8 in, 1 out]
                                n707 = call "Advanced Serial.vi"("Write"=TRUE ("write"), "string to write"=w1142) -> ()  [unwired: 3 in, 7 out]
                                }
                                frame #1 {
                                n708 = while {
                                tunnel: [w1160] -> w1146
                                tunnel: [w1159] -> w1152
                                tunnel: [w1155] -> w1147
                                tunnel: [w1158] -> w1148
                                tunnel: [w1157] -> w1149
                                tunnel: [w1156] -> w1150
                                tunnel: [w1155] -> w1153
                                stop <- w1161 stop-if-true
                                n709 = call "Advanced Serial.vi"() -> ("RTD-02 (ºC)"=w1157:sgl, "RTD-01 (ºC)"=w1158:sgl, "vacuo (mBar)"=w1159:dbl, "P02 (Bar)"=w1155:dbl, "RTD-chamber (ºC)"=w1156:sgl, "P01 (Bar)"=w1160:dbl, "32bytes"=w1161:bool)  [unwired: 5 in]
                                }
                                n710 = Wait Until Next ms Multiple(millisecond multiple=u32 5) -> ()  [unwired: 1 out]
                                n711 = local write "Vol01"(w1146) -> ()
                                n712 = local write "Vol02"(w1153) -> ()
                                n713 = local write "Pcin"(w1153) -> ()
                                n714 = Merge Signals(w1146, w1147, w1152, w1148, w1149, w1150) -> (w1151:dynamicdata)
                                n715 = local write "graph_completo"(w1151) -> ()
                                }
                                frame #2 {
                                n716 = call "data2byte.vi"("argument"=0.0, "new function"=5.0) -> ("protocol"=w1162:string)  [unwired: 8 in, 1 out]
                                n717 = call "Advanced Serial.vi"("Write"=TRUE ("write"), "string to write"=w1162) -> ()  [unwired: 3 in, 7 out]
                                }
                                frame #3 {
                                n718 = Wait Until Next ms Multiple(millisecond multiple=u32 5) -> ()  [unwired: 1 out]
                                }
                                }
                                }
                                }
                              }
                              frame #1 {
                                n719 = call "data2byte.vi"("argument"=1.0, "new function"=5.0) -> ("protocol"=w1170:string)  [unwired: 8 in, 1 out]
                                n720 = local write "descarga 2"(FALSE ("descarga")) -> ()
                                n721 = call "Advanced Serial.vi"("Write"=TRUE ("write"), "string to write"=w1170) -> ()  [unwired: 3 in, 7 out]
                              }
                              frame #2 {
                                n722 = while {
                                tunnel: [w1187] -> w1181
                                tunnel: [w1186] -> w1174
                                tunnel: [w1182] -> w1180
                                tunnel: [w1185] -> w1179
                                tunnel: [w1184] -> w1178
                                tunnel: [w1183] -> w1177
                                tunnel: [w1182] -> w1175
                                stop <- w1188 stop-if-true
                                n723 = call "Advanced Serial.vi"() -> ("RTD-02 (ºC)"=w1184:sgl, "RTD-01 (ºC)"=w1185:sgl, "vacuo (mBar)"=w1186:dbl, "P02 (Bar)"=w1182:dbl, "RTD-chamber (ºC)"=w1183:sgl, "P01 (Bar)"=w1187:dbl, "32bytes"=w1188:bool)  [unwired: 5 in]
                                }
                                n724 = local write "Vol01"(w1181) -> ()
                                n725 = local write "Vol02"(w1175) -> ()
                                n726 = Merge Signals(w1181, w1180, w1174, w1179, w1178, w1177) -> (w1176:dynamicdata)
                                n727 = Multiply(x=w1174, y=0.001) -> (x*y=w1172:dbl)
                                n728 = local write "graph_completo"(w1176) -> ()
                                n729 = local write "Pcin"(w1172) -> ()
                              }
                            }
                          }
                          frame True {
                            n730 = property on="descarga 2" class="Bool (strict)"() -> ("Value"=w1190:bool)  [unwired: 2 in, 2 out]
                            n731 = case shown="True" w1190 {
                              selector: w1190 -> [_ w1293]
                              tunnel: w1189 -> [_ w1294]
                              frame False {
                                n732 = property on="clear sample" class="Bool (strict)"() -> ("Value"=w1191:bool)  [unwired: 2 in, 2 out]
                                n733 = case shown="True" w1191 {
                                frame False {
                                n734 = while {
                                tunnel: [w1218] -> w1193
                                tunnel: [w1217] -> w1200
                                tunnel: [w1213] -> w1194
                                tunnel: [w1216] -> w1195
                                tunnel: [w1215] -> w1196
                                tunnel: [w1214] -> w1197
                                tunnel: [w1213] -> w1199
                                stop <- w1219 stop-if-true
                                n735 = call "Advanced Serial.vi"() -> ("RTD-02 (ºC)"=w1215:sgl, "RTD-01 (ºC)"=w1216:sgl, "vacuo (mBar)"=w1217:dbl, "P02 (Bar)"=w1213:dbl, "RTD-chamber (ºC)"=w1214:sgl, "P01 (Bar)"=w1218:dbl, "32bytes"=w1219:bool)  [unwired: 5 in]
                                }
                                n736 = Tick Count (ms)() -> (millisecond timer value=w1211:u32)
                                n737 = Build Array(w1211) -> (w1205:u32[])
                                n738 = property on="cont_vacuo" class="Arr (strict)"() -> ("Value"=w1212:u32[])  [unwired: 2 in, 2 out]
                                n739 = Insert Into Array(array=w1212, new element=w1205) -> (w1206:u32[])  [unwired: 1 in]
                                "cont_vacuo" <- w1206
                                n740 = local write "Vol01"(w1193) -> ()
                                n741 = local write "Vol02"(w1199) -> ()
                                n742 = Array Max & Min(array=w1206) -> (max value=w1210:u32, min value=w1209:u32)  [unwired: 2 out]
                                n743 = Subtract(x=w1210, y=w1209) -> (x-y=w1207:u32)
                                n744 = Multiply(x=w1200, y=0.001) -> (x*y=w1192:dbl)
                                n745 = local write "Pcin"(w1192) -> ()
                                n746 = Divide(x=w1207, y=1000.0) -> (x/y=w1204:dbl)
                                "time" <- w1204
                                n747 = Merge Signals(w1193, w1194, w1200, w1195, w1196, w1197, w1192) -> (w1198:dynamicdata)
                                n748 = local write "graph_completo"(w1198) -> ()
                                n749 = Greater?(x=w1204, y="t-vacuo (s)") -> (0:w1202:bool)
                                n750 = case shown="True" w1202 {
                                selector: w1202 -> [_ w1224]
                                frame False {
                                n751 = call "data2byte.vi"("argument"=1.0 ("number"), "new function"=5.0) -> ("protocol"=w1220:string)  [unwired: 8 in, 1 out]
                                n752 = call "Advanced Serial.vi"("Write"=TRUE ("write"), "string to write"=w1220) -> ()  [unwired: 3 in, 7 out]
                                }
                                frame True {
                                n753 = flat-sequence {
                                tunnel: w1224 -> [w1231]
                                frame #0 {
                                n754 = local write "descarga 2"(w1231) -> ()
                                n755 = local write "time-loop"(1.0 ("time-loop")) -> ()
                                n756 = local write "Pvol2 total"(dbl[] [] ("output array 2")) -> ()
                                n757 = local write "cont_desc min"(dbl[] [] ("output array 2")) -> ()
                                n758 = local write "dP/dt"(dbl[] [] ("output array 2")) -> ()
                                n759 = local write "time (min) 3"(dbl[] [] ("output array 2")) -> ()
                                n760 = local write "cont_vacuo"(u32[] [] ("output array 2")) -> ()
                                }
                                frame #1 {
                                n761 = call "data2byte.vi"("argument"=0.0 ("number"), "new function"=5.0) -> ("protocol"=w1232:string)  [unwired: 8 in, 1 out]
                                n762 = call "Advanced Serial.vi"("Write"=TRUE ("write"), "string to write"=w1232) -> ()  [unwired: 3 in, 7 out]
                                }
                                frame #2 {
                                n763 = while {
                                tunnel: [w1270] -> w1250
                                tunnel: [w1269] -> w1246
                                tunnel: [w1265] -> w1249
                                tunnel: [w1268] -> w1241
                                tunnel: [w1267] -> w1239
                                tunnel: [w1266] -> w1240
                                tunnel: [w1265] -> w1247
                                stop <- w1271 stop-if-true
                                n764 = call "Advanced Serial.vi"() -> ("RTD-02 (ºC)"=w1267:sgl, "RTD-01 (ºC)"=w1268:sgl, "vacuo (mBar)"=w1269:dbl, "P02 (Bar)"=w1265:dbl, "RTD-chamber (ºC)"=w1266:sgl, "P01 (Bar)"=w1270:dbl, "32bytes"=w1271:bool)  [unwired: 5 in]
                                }
                                n765 = property on="Save Discharge" class="Bool (strict)"() -> ("Value"=w1243:bool)  [unwired: 2 in, 2 out]
                                n766 = local write "Vol01"(w1250) -> ()
                                n767 = local write "Vol02"(w1247) -> ()
                                n768 = property on="Ch Max" class="Bool (strict)"() -> ("Value"=w1244:bool)  [unwired: 2 in, 2 out]
                                n769 = And(x=w1244, y=w1243) -> (x .and. y?=w1238:bool)
                                n770 = Multiply(x=w1246, y=0.001) -> (x*y=w1242:dbl)
                                n771 = property on="ISO Start" class="Bool (strict)"() -> ("Value"=w1236:bool)  [unwired: 2 in, 2 out]
                                n772 = local write "Pcin"(w1242) -> ()
                                n773 = Or(x=w1238, y=w1236) -> (x .or. y?=w1237:bool)
                                n774 = Merge Signals(w1250, w1249, w1246, w1241, w1239, w1240, w1242) -> (w1248:dynamicdata)
                                n775 = case shown="True" w1237 {
                                tunnel: w1242 -> [_ w1257]
                                tunnel: w1241 -> [_ w1256]
                                tunnel: w1240 -> [_ w1255]
                                tunnel: w1239 -> [_ w1254]
                                frame False {
                                }
                                frame True {
                                w1253 = "\t"
                                w1259 = i16 4 ("precision (6)")
                                n776 = Number To Fractional String(number=w1257, precision (6)=w1259) -> (F-format string=w1252:string)  [unwired: 2 in]
                                n777 = Number To Fractional String(number=w1256, precision (6)=w1259) -> (F-format string=w1262:string)  [unwired: 2 in]
                                n778 = Number To Fractional String(number=w1254, precision (6)=w1259) -> (F-format string=w1258:string)  [unwired: 2 in]
                                n779 = Number To Fractional String(number=w1255, precision (6)=w1259) -> (F-format string=w1261:string)  [unwired: 2 in]
                                n780 = Concatenate Strings(w1252, w1253, w1262, w1253, w1261, w1253, w1258, "\r\n") -> (w1264:string)
                                n781 = property on="pathISO" class="Path"() -> ("Value"=w1263:path)  [unwired: 2 in, 2 out]
                                n782 = call "write_file.vi"("text"=w1264, "file path (use dialog)"=w1263) -> ()  [unwired: 10 in]
                                }
                                }
                                n783 = local write "graph_completo"(w1248) -> ()
                                n784 = Wait Until Next ms Multiple(millisecond multiple=u32 5) -> ()  [unwired: 1 out]
                                }
                                frame #3 {
                                n785 = call "data2byte.vi"("argument"=1.0 ("number"), "new function"=2.0) -> ("protocol"=w1272:string)  [unwired: 8 in, 1 out]
                                n786 = call "Advanced Serial.vi"("Write"=TRUE ("write"), "string to write"=w1272) -> ()  [unwired: 3 in, 7 out]
                                }
                                frame #4 {
                                n787 = while {
                                tunnel: [w1289] -> w1283
                                tunnel: [w1288] -> w1277
                                tunnel: [w1284] -> w1282
                                tunnel: [w1287] -> w1281
                                tunnel: [w1286] -> w1280
                                tunnel: [w1285] -> w1279
                                tunnel: [w1284] -> w1276
                                stop <- w1290 stop-if-true
                                n788 = call "Advanced Serial.vi"() -> ("RTD-02 (ºC)"=w1286:sgl, "RTD-01 (ºC)"=w1287:sgl, "vacuo (mBar)"=w1288:dbl, "P02 (Bar)"=w1284:dbl, "RTD-chamber (ºC)"=w1285:sgl, "P01 (Bar)"=w1289:dbl, "32bytes"=w1290:bool)  [unwired: 5 in]
                                }
                                n789 = local write "Vol01"(w1283) -> ()
                                n790 = local write "Pcin"(w1276) -> ()
                                n791 = local write "Vol02"(w1276) -> ()
                                n792 = Merge Signals(w1283, w1282, w1277, w1281, w1280, w1279, w1276) -> (w1278:dynamicdata)
                                n793 = local write "graph_completo"(w1278) -> ()
                                }
                                }
                                }
                                }
                                }
                                frame True {
                                }
                                }
                              }
                              frame True {
                                n794 = flat-sequence {
                                tunnel: w1293 -> [w1299]
                                tunnel: w1294 -> [w1296]
                                tunnel: [w1296] -> w1292
                                tunnel: [w1299] -> w1291
                                tunnel: w1292 -> [w1367]
                                tunnel: w1291 -> [w1366]
                                frame #0 {
                                n795 = property on="x >= y? 2" class="Bool (strict)"() -> ("Value"=w1298:bool)  [unwired: 2 in, 2 out]
                                n796 = property on="time-loop" class="DigNum (strict)"() -> ("Value"=w1297:dbl)  [unwired: 2 in, 2 out]
                                n797 = case shown="True" w1298 {
                                tunnel: w1297 -> [_ w1334]
                                frame False {
                                }
                                frame True {
                                n798 = Increment(x=w1334) -> (x+1=→"time-loop":dbl)
                                n799 = property on="Numeric" class="DigNum (strict)"() -> ("Value"=w1328:dbl)  [unwired: 2 in, 2 out]
                                n800 = local write "time 2"(dbl[] [] ("output array 2")) -> ()
                                n801 = local write "cont_desc"(dbl[] [] ("output array 2")) -> ()
                                n802 = local write "Pvol2"(dbl[] [] ("output array 2")) -> ()
                                n803 = Less Or Equal?(x=w1328, y=1.09) -> (x <= y?=w1332:bool)
                                n804 = property on="slop" class="Bool (strict)"() -> ("Value"=w1331:bool)  [unwired: 2 in, 2 out]
                                n805 = And(x=w1332, y=w1331) -> (x .and. y?=w1330:bool)
                                n806 = property on="N 1bar" class="DigNum (strict)"() -> ("Value"=w1329:i32)  [unwired: 2 in, 2 out]
                                n807 = case shown="True" w1330 {
                                tunnel: w1329 -> [_ w1343]
                                frame False {
                                }
                                frame True {
                                n808 = Increment(x=w1343) -> (x+1=w1342:i32)
                                "N 1bar" <- w1342
                                n809 = Less Or Equal?(x=w1342, y=3) -> (x <= y?=w1339:bool)
                                n810 = local write "descarga 2"(w1339) -> ()
                                n811 = Not(x=w1339) -> (.not. x?=w1340:bool)
                                n812 = local write "clear sample"(w1340) -> ()
                                }
                                }
                                }
                                }
                                n813 = local write "Chamber"(w1296) -> ()
                                n814 = property on="Kinetic Save" class="Bool (strict)"() -> ("Value"=w1295:bool)  [unwired: 2 in, 2 out]
                                n815 = case shown="True" w1295 {
                                frame False {
                                }
                                frame True {
                                w1305 = "\t"
                                w1302 = i16 4 ("precision (6)")
                                n816 = while {
                                tunnel: [w1326] -> w1316
                                tunnel: [w1325] -> w1314
                                tunnel: [w1324] -> w1312
                                tunnel: [w1322] -> w1310
                                tunnel: [w1323] -> w1308
                                stop <- w1327 stop-if-true
                                n817 = call "Advanced Serial.vi"() -> ("RTD-02 (ºC)"=w1323:sgl, "RTD-01 (ºC)"=w1324:sgl, "P02 (Bar)"=w1325:dbl, "RTD-chamber (ºC)"=w1322:sgl, "P01 (Bar)"=w1326:dbl, "32bytes"=w1327:bool)  [unwired: 5 in, 1 out]
                                }
                                n818 = property on="Pcin" class="Slide (strict)"() -> ("Value"=w1300:dbl)  [unwired: 2 in, 2 out]
                                n819 = Number To Fractional String(number=w1300, precision (6)=w1302) -> (F-format string=w1303:string)  [unwired: 2 in]
                                n820 = Number To Fractional String(number=w1316, precision (6)=w1302) -> (F-format string=w1318:string)  [unwired: 2 in]
                                n821 = Number To Fractional String(number=w1314, precision (6)=w1302) -> (F-format string=w1317:string)  [unwired: 2 in]
                                n822 = Number To Fractional String(number=w1312, precision (6)=w1302) -> (F-format string=w1313:string)  [unwired: 2 in]
                                n823 = Number To Fractional String(number=w1310, precision (6)=w1302) -> (F-format string=w1311:string)  [unwired: 2 in]
                                n824 = Number To Fractional String(number=w1308, precision (6)=w1302) -> (F-format string=w1309:string)  [unwired: 2 in]
                                n825 = Get Date/Time String(want seconds? (F)=TRUE) -> (date string=w1321:string, time string=w1319:string)  [unwired: 2 in]
                                n826 = Concatenate Strings(w1321, "-" ("string"), w1319, w1305, w1318, w1305, "-" ("string"), w1305, w1317, w1305, w1313, w1305, w1311, w1305, w1309, w1305, w1303, "\r\n") -> (w1307:string)
                                n827 = property on="path" class="Path"() -> ("Value"=w1301:path)  [unwired: 2 in, 2 out]
                                n828 = call "write_file.vi"("text"=w1307, "file path (use dialog)"=w1301) -> ()  [unwired: 10 in]
                                }
                                }
                                }
                                frame #1 {
                                n829 = Build Array(w1367) -> (w1389:dbl[])
                                n830 = Build Array(w1367) -> (w1372:dbl[])
                                n831 = property on="time-loop" class="DigNum (strict)"() -> ("Value"=w1355:dbl)  [unwired: 2 in, 2 out]
                                n832 = Tick Count (ms)() -> (millisecond timer value=w1396:u32)
                                n833 = Tick Count (ms)() -> (millisecond timer value=w1375:u32)
                                n834 = Build Array(w1396) -> (w1390:u32[])
                                n835 = Build Array(w1375) -> (w1381:u32[])
                                n836 = property on="Pvol2" class="Arr (strict)"() -> ("Value"=w1388:dbl[])  [unwired: 2 in, 2 out]
                                n837 = property on="time (min) 3" class="Arr (strict)"() -> ("Value"=w1370:dbl[])  [unwired: 2 in, 2 out]
                                n838 = property on="cont_desc min" class="Arr (strict)"() -> ("Value"=w1374:dbl[])  [unwired: 2 in, 2 out]
                                n839 = property on="Pvol2 total" class="Arr (strict)"() -> ("Value"=w1373:dbl[])  [unwired: 2 in, 2 out]
                                n840 = Multiply(x=w1355, y=10.0 ("time-fit (s)")) -> (x*y=w1356:dbl)
                                n841 = Insert Into Array(array=w1388, new element=w1389) -> (w1347:dbl[])  [unwired: 1 in]
                                "Pvol2" <- w1347
                                n842 = Insert Into Array(array=w1373, new element=w1372) -> (w1369:dbl[])  [unwired: 1 in]
                                "Pvol2 total" <- w1369
                                n843 = Insert Into Array(array=w1374, new element=w1381) -> (w1380:dbl[])  [unwired: 1 in]
                                "cont_desc min" <- w1380
                                n844 = property on="cont_desc" class="Arr (strict)"() -> ("Value"=w1397:dbl[])  [unwired: 2 in, 2 out]
                                n845 = Insert Into Array(array=w1397, new element=w1390) -> (w1391:dbl[])  [unwired: 1 in]
                                "cont_desc" <- w1391
                                n846 = Array Max & Min(array=w1380) -> (max value=w1376:dbl, min value=w1377:dbl)  [unwired: 2 out]
                                n847 = Subtract(x=w1376, y=w1377) -> (x-y=w1379:dbl)
                                n848 = Array Max & Min(array=w1391) -> (max value=w1395:dbl, min value=w1394:dbl)  [unwired: 2 out]
                                n849 = Divide(x=w1379, y=60000.0) -> (x/y=w1359:dbl)
                                "time (min) 2" <- w1359
                                n850 = Subtract(x=w1395, y=w1394) -> (x-y=w1392:dbl)
                                n851 = Build Array(w1359) -> (w1371:dbl[])
                                n852 = call <vilib>:"Derivative x(t) PtByPt.vi"("initialize"=w1366, "dt"=w1359, "x"=w1367) -> ("dx/dt"=w1354:dbl)  [unwired: 1 in, 1 out]
                                "dp/dt 2" <- w1354
                                n853 = Divide(x=w1392, y=1000.0) -> (x/y=w1362:dbl)
                                n854 = Insert Into Array(array=w1370, new element=w1371) -> (w1368:dbl[])  [unwired: 1 in]
                                "time (min) 3" <- w1368
                                n855 = Greater Or Equal?(x=w1362, y=w1356) -> (x >= y?=w1358:bool)
                                "x >= y? 2" <- w1358
                                n856 = Build Array(w1362) -> (w1386:dbl[])
                                n857 = Bundle("Value"=w1368, "Value"=w1369) -> (w1353:cluster{"Value":dbl[], "Value":dbl[]})  [unwired: 1 in]
                                n858 = Build Array(w1354) -> (w1365:dbl[])
                                n859 = property on="time 2" class="Arr (strict)"() -> ("Value"=w1387:dbl[])  [unwired: 2 in, 2 out]
                                n860 = property on="dP/dt" class="Arr (strict)"() -> ("Value"=w1364:dbl[])  [unwired: 2 in, 2 out]
                                n861 = Insert Into Array(array=w1387, new element=w1386) -> (w1346:dbl[])  [unwired: 1 in]
                                "time 2" <- w1346
                                n862 = Insert Into Array(array=w1364, new element=w1365) -> (w1363:dbl[])  [unwired: 1 in]
                                "dP/dt" <- w1363
                                n863 = call <vilib>:"General Polynomial Fit.vi"("Y"=w1347, "polynomial order"=0, "X"=w1346) -> ("Best Polynomial Fit"=w1348:dbl[], "Polynomial Coefficients"=w1349:dbl[])  [unwired: 9 in, 2 out]
                                n864 = call <vilib>:"Linear Fit.vi"("Y"=w1347, "X"=w1346) -> ("Best Linear Fit"=w1383:dbl[], "slope"=w1361:dbl)  [unwired: 9 in, 3 out]
                                "slope 2" <- w1361
                                n865 = Bundle("Value"=w1346, "Value"=w1347) -> (w1384:cluster{"Value":dbl[], "Value":dbl[]})  [unwired: 1 in]
                                n866 = Bundle("Value"=w1368, "Value"=w1363) -> (w1352:cluster{"Value":dbl[], "Value":dbl[]})  [unwired: 1 in]
                                n867 = Build Array(w1353, w1352) -> (→"fit-all 2":cluster{"Value":dbl[], "Value":dbl[]}[])
                                n868 = Bundle("Value"=w1346, "Best Polynomial Fit"=w1348) -> (w1350:T8)  [unwired: 1 in]
                                n869 = Index Array(array=w1349) -> (element=w1344:dbl)  [unwired: 1 in]
                                n870 = local write "Pfit"(w1344) -> ()
                                n871 = Absolute Value(x=w1361) -> (abs(x)=w1360:dbl)
                                n872 = Bundle("Value"=w1346, "Best Linear Fit"=w1383) -> (w1385:cluster{"Value":dbl[], "Best Linear Fit":dbl[]})  [unwired: 1 in]
                                n873 = case shown="True" w1358 {
                                tunnel: w1360 -> [_ w1409]
                                tunnel: w1359 -> [_ w1407]
                                tunnel: w1354 -> [_ w1404]
                                tunnel: w1344 -> [_ w1399]
                                frame False {
                                }
                                frame True {
                                n874 = Less Or Equal?(x=w1404, y="dp/dt min 2") -> (x <= y?=w1403:bool)
                                n875 = Greater Or Equal?(x=w1407, y="total Time(min) 2") -> (x >= y?=w1408:bool)
                                n876 = Less Or Equal?(x=w1409, y="Mininum Slope 2") -> (x <= y?=w1406:bool)
                                "slop" <- w1406
                                n877 = Or(x=w1406, y=w1403) -> (x .or. y?=w1402:bool)
                                n878 = Or(x=w1402, y=w1408) -> (x .or. y?=w1410:bool)
                                n879 = case shown="True" w1410 {
                                tunnel: w1399 -> [_ w1416]
                                frame False {
                                n880 = local write "estado"(TRUE ("estado")) -> ()
                                n881 = local write "descarga 2"(TRUE ("descarga")) -> ()
                                }
                                frame True {
                                n882 = flat-sequence {
                                tunnel: [w1418] -> w1417
                                tunnel: w1416 -> [w1418]
                                tunnel: [w1420] -> w1415
                                tunnel: [w1419] -> w1414
                                tunnel: [w1418] -> w1413
                                tunnel: w1417 -> [w1430]
                                tunnel: w1415 -> [w1429]
                                tunnel: w1414 -> [w1428]
                                tunnel: w1413 -> [w1427]
                                frame #0 {
                                n883 = call "data2byte.vi"("argument"=0.0 ("number"), "new function"=2.0) -> ("protocol"=w1421:string)  [unwired: 8 in, 1 out]
                                n884 = property on="Save Discharge" class="Bool (strict)"() -> ("Value"=w1425:bool)  [unwired: 2 in, 2 out]
                                n885 = call "Advanced Serial.vi"("Write"=TRUE ("write"), "string to write"=w1421) -> ()  [unwired: 3 in, 7 out]
                                n886 = property on="Ch Max" class="Bool (strict)"() -> ("Value"=w1426:bool)  [unwired: 2 in, 2 out]
                                n887 = And(x=w1426, y=w1425) -> (x .and. y?=w1420:bool)
                                n888 = property on="ISO Start" class="Bool (strict)"() -> ("Value"=w1419:bool)  [unwired: 2 in, 2 out]
                                }
                                frame #1 {
                                n889 = case shown="True" w1429 {
                                tunnel: w1427 -> [_ w1431]
                                frame False {
                                }
                                frame True {
                                n890 = flat-sequence {
                                tunnel: [w1433] -> w1432
                                tunnel: w1432 -> [w1436]
                                tunnel: w1431 -> [w1435]
                                frame #0 {
                                n891 = property on="Set ChM" class="DigNum (strict)"() -> ("Value"=w1434:dbl)  [unwired: 2 in, 2 out]
                                n892 = Increment(x=w1434) -> (x+1=w1433:dbl)
                                n893 = local write "Set ChM"(w1433) -> ()
                                }
                                frame #1 {
                                w1443 = i16 0 ("precision (6)")
                                w1437 = "\t"
                                n894 = property on="Cycles" class="DigNum (strict)"() -> ("Value"=w1442:dbl)  [unwired: 2 in, 2 out]
                                n895 = Number To Fractional String(number=w1435, precision (6)=i16 4) -> (F-format string=w1438:string)  [unwired: 2 in]
                                n896 = Number To Fractional String(number=w1442, precision (6)=w1443) -> (F-format string=w1441:string)  [unwired: 2 in]
                                n897 = Number To Fractional String(number=w1436, precision (6)=w1443) -> (F-format string=w1440:string)  [unwired: 2 in]
                                n898 = Concatenate Strings(w1441, w1437, w1440, w1437, "==>", w1437, w1438, w1437) -> (w1446:string)
                                n899 = property on="pathISO" class="Path"() -> ("Value"=w1445:path)  [unwired: 2 in, 2 out]
                                n900 = call "write_file.vi"("text"=w1446, "file path (use dialog)"=w1445) -> ()  [unwired: 10 in]
                                }
                                }
                                }
                                }
                                n901 = case shown="True" w1428 {
                                tunnel: w1430 -> [_ w1448]
                                frame False {
                                }
                                frame True {
                                n902 = flat-sequence {
                                tunnel: [w1452] -> w1449
                                tunnel: w1448 -> [w1452]
                                tunnel: [w1450] -> w1447
                                tunnel: w1449 -> [w1456]
                                tunnel: w1447 -> [w1453]
                                frame #0 {
                                n903 = property on="Set ISO" class="DigNum (strict)"() -> ("Value"=w1451:dbl)  [unwired: 2 in, 2 out]
                                n904 = Increment(x=w1451) -> (x+1=w1450:dbl)
                                n905 = local write "Set ISO"(w1450) -> ()
                                }
                                frame #1 {
                                w1461 = i16 0 ("precision (6)")
                                w1454 = "\t"
                                n906 = property on="Cycles" class="DigNum (strict)"() -> ("Value"=w1460:dbl)  [unwired: 2 in, 2 out]
                                n907 = Number To Fractional String(number=w1456, precision (6)=i16 4) -> (F-format string=w1455:string)  [unwired: 2 in]
                                n908 = Number To Fractional String(number=w1460, precision (6)=w1461) -> (F-format string=w1459:string)  [unwired: 2 in]
                                n909 = Number To Fractional String(number=w1453, precision (6)=w1461) -> (F-format string=w1458:string)  [unwired: 2 in]
                                n910 = Concatenate Strings(w1459, w1454, w1458, w1454, "==>", w1454, w1455, w1454) -> (w1464:string)
                                n911 = property on="pathISO" class="Path"() -> ("Value"=w1463:path)  [unwired: 2 in, 2 out]
                                n912 = call "write_file.vi"("text"=w1464, "file path (use dialog)"=w1463) -> ()  [unwired: 10 in]
                                }
                                }
                                }
                                }
                                }
                                frame #2 {
                                n913 = local write "time-loop"(1.0 ("time-loop")) -> ()
                                n914 = local write "descarga 2"(FALSE ("descarga")) -> ()
                                n915 = local write "dP/dt"(dbl[] [] ("output array 2")) -> ()
                                n916 = local write "Pvol2 total"(dbl[] [] ("output array 2")) -> ()
                                n917 = local write "cont_desc min"(dbl[] [] ("output array 2")) -> ()
                                n918 = local write "time (min) 3"(dbl[] [] ("output array 2")) -> ()
                                }
                                }
                                }
                                }
                                "Numeric" <- w1399
                                }
                                }
                                n919 = Build Array(w1385, w1384, w1350) -> (→"slop01 2":T3)
                                "descarga 2" <- TRUE
                                }
                                }
                              }
                            }
                          }
                        }
                      }
                    }
                  }
                }
              }
            }
          }
        }
      }
      frame #4 {
        n920 = case shown="True" "clear sample" {
          selector: "clear sample" -> [_ w1476]
          tunnel: [FALSE w1474] -> w1471
          frame False {
          }
          frame True {
            n921 = property on="Cycles" class="DigNum (strict)"() -> ("Value"=w1475:dbl)  [unwired: 2 in, 2 out]
            n922 = property on="N cycles" class="DigNum (strict)"() -> ("Value"=w1477:dbl)  [unwired: 2 in, 2 out]
            n923 = Greater Or Equal?(x=w1477, y=w1475) -> (x >= y?=w1478:bool)
            n924 = case shown="True" w1478 {
              selector: w1478 -> [_ w1496]
              tunnel: w1476 -> [w1480 _]
              tunnel: [w1479 w1486] -> w1474
              frame False {
                n925 = flat-sequence {
                  tunnel: [w1482] -> w1481
                  tunnel: w1480 -> [w1482]
                  tunnel: w1481 -> [w1484]
                  tunnel: [TRUE] -> w1479
                  frame #0 {
                    w1483 = FALSE ("Ch Max")
                    n926 = local write "Ch Max"(w1483) -> ()
                    n927 = local write "Save Discharge"(w1483) -> ()
                    n928 = local write "PCS"(w1483) -> ()
                    n929 = local write "Kinetic Save"(w1483) -> ()
                    n930 = local write "Discharge"(w1483) -> ()
                  }
                  frame #1 {
                    n931 = local write "close All"(w1484) -> ()
                  }
                  frame #2 {
                  }
                }
              }
              frame True {
                n932 = flat-sequence {
                  tunnel: w1496 -> [w1499]
                  tunnel: [w1499] -> w1492
                  tunnel: [w1525] -> w1494
                  tunnel: w1492 -> [w1525]
                  tunnel: [w1515] -> w1489
                  tunnel: w1494 -> [w1529]
                  tunnel: [w1529] -> w1493
                  tunnel: ["t-vacuo (s) clean"] -> w1490
                  tunnel: w1489 -> [w1527]
                  tunnel: [w1527] -> w1488
                  tunnel: w1493 -> [w1536]
                  tunnel: [w1536] -> w1495
                  tunnel: [w1535] -> w1491
                  tunnel: w1490 -> [w1535]
                  tunnel: w1488 -> [w1534]
                  tunnel: [w1534] -> w1487
                  tunnel: w1495 -> [_]
                  tunnel: w1491 -> [w1539]
                  tunnel: w1487 -> [w1538]
                  tunnel: [w1537] -> w1486
                  frame #0 {
                    n933 = stacked-sequence {
                      tunnel: 0.0 ("number") -> [w1501 _ w1504 w1508 _]
                      tunnel: TRUE ("write") -> [w1500 _ w1505 w1509 _]
                      frame #0 {
                        n934 = call "data2byte.vi"("argument"=w1501, "new function"=1.0) -> ("protocol"=w1502:string)  [unwired: 8 in, 1 out]
                        n935 = call "Advanced Serial.vi"("Write"=w1500, "string to write"=w1502) -> ()  [unwired: 3 in, 7 out]
                      }
                      frame #1 {
                      }
                      frame #2 {
                        n936 = call "data2byte.vi"("argument"=w1504, "new function"=3.0) -> ("protocol"=w1506:string)  [unwired: 8 in, 1 out]
                        n937 = call "Advanced Serial.vi"("Write"=w1505, "string to write"=w1506) -> ()  [unwired: 3 in, 7 out]
                      }
                      frame #3 {
                        n938 = call "data2byte.vi"("argument"=w1508, "new function"=4.0) -> ("protocol"=w1510:string)  [unwired: 8 in, 1 out]
                        n939 = call "Advanced Serial.vi"("Write"=w1509, "string to write"=w1510) -> ()  [unwired: 3 in, 7 out]
                      }
                      frame #4 {
                      }
                    }
                  }
                  frame #1 {
                    n940 = Tick Count (ms)() -> (millisecond timer value=w1517:u32)
                    n941 = call "data2byte.vi"("argument"=1.0 ("number"), "new function"=2.0) -> ("protocol"=w1512:string)  [unwired: 8 in, 1 out]
                    n942 = Build Array(w1517) -> (w1523:u32[])
                    n943 = property on="cont_vacuo 2" class="Arr (strict)"() -> ("Value"=w1516:u32[])  [unwired: 2 in, 2 out]
                    n944 = call "Advanced Serial.vi"("Write"=TRUE ("write"), "string to write"=w1512) -> ()  [unwired: 3 in, 7 out]
                    n945 = Insert Into Array(array=w1516, new element=w1523) -> (w1522:u32[])  [unwired: 1 in]
                    "cont_vacuo 2" <- w1522
                    n946 = Array Max & Min(array=w1522) -> (max value=w1518:u32, min value=w1519:u32)  [unwired: 2 out]
                    n947 = Subtract(x=w1518, y=w1519) -> (x-y=w1521:u32)
                    n948 = Divide(x=w1521, y=1000.0) -> (x/y=w1515:dbl)
                    "time 3" <- w1515
                  }
                  frame #2 {
                    n949 = Wait Until Next ms Multiple(millisecond multiple=u32 5) -> ()  [unwired: 1 out]
                  }
                  frame #3 {
                    n950 = call "data2byte.vi"("argument"=1.0 ("number"), "new function"=5.0) -> ("protocol"=w1530:string)  [unwired: 8 in, 1 out]
                    n951 = call "Advanced Serial.vi"("Write"=TRUE ("write"), "string to write"=w1530) -> ()  [unwired: 3 in, 7 out]
                  }
                  frame #4 {
                    n952 = Greater?(x=w1538, y=w1539) -> (0:w1540:bool)
                    n953 = case shown="True" w1540 {
                      selector: w1540 -> [_ w1555]
                      tunnel: [FALSE ("write") w1547] -> w1537
                      frame False {
                        n954 = call "data2byte.vi"("argument"=1.0 ("number"), "new function"=5.0) -> ("protocol"=w1545:string)  [unwired: 8 in, 1 out]
                        n955 = call "Advanced Serial.vi"("Write"=TRUE ("write"), "string to write"=w1545) -> ()  [unwired: 3 in, 7 out]
                      }
                      frame True {
                        n956 = flat-sequence {
                          tunnel: w1555 -> [w1556]
                          tunnel: [w1556] -> w1550
                          tunnel: [w1568] -> w1551
                          tunnel: w1550 -> [w1568]
                          tunnel: [w1569] -> w1552
                          tunnel: w1551 -> [w1569]
                          tunnel: [w1575] -> w1553
                          tunnel: w1552 -> [w1575]
                          tunnel: [w1584] -> w1554
                          tunnel: w1553 -> [w1584]
                          tunnel: [w1576] -> w1549
                          tunnel: w1554 -> [w1609]
                          tunnel: [w1610] -> w1548
                          tunnel: w1549 -> [w1608]
                          tunnel: [w1607] -> w1546
                          frame #0 {
                            n957 = local write "N 1bar"(0 ("N 1bar")) -> ()
                            n958 = local write "time-loop"(1.0 ("time-loop")) -> ()
                            n959 = local write "cont_desc min"(dbl[] [] ("output array 2")) -> ()
                            n960 = local write "time (min) 3"(dbl[] [] ("output array 2")) -> ()
                            n961 = local write "Pvol2 total"(dbl[] [] ("output array 2")) -> ()
                            n962 = local write "dP/dt"(dbl[] [] ("output array 2")) -> ()
                            n963 = local write "cont_vacuo 2"(u32[] [] ("output array 2")) -> ()
                          }
                          frame #1 {
                            n964 = call "data2byte.vi"("argument"=0.0 ("number"), "new function"=5.0) -> ("protocol"=w1567:string)  [unwired: 8 in, 1 out]
                            n965 = call "Advanced Serial.vi"("Write"=TRUE ("write"), "string to write"=w1567) -> ()  [unwired: 3 in, 7 out]
                          }
                          frame #2 {
                            n966 = Wait Until Next ms Multiple(millisecond multiple=u32 5) -> ()  [unwired: 1 out]
                          }
                          frame #3 {
                            n967 = call "data2byte.vi"("argument"=0.0 ("number"), "new function"=2.0) -> ("protocol"=w1571:string)  [unwired: 8 in, 1 out]
                            n968 = call "Advanced Serial.vi"("Write"=TRUE ("write"), "string to write"=w1571) -> ()  [unwired: 3 in, 7 out]
                          }
                          frame #4 {
                            n969 = while {
                              tunnel: [w1605] -> w1594
                              tunnel: [w1604] -> w1590
                              tunnel: [w1600] -> w1593
                              tunnel: [w1603] -> w1587
                              tunnel: [w1602] -> w1585
                              tunnel: [w1601] -> w1586
                              tunnel: [w1600] -> w1591
                              stop <- w1606 stop-if-true
                              n970 = call "Advanced Serial.vi"() -> ("RTD-02 (ºC)"=w1602:sgl, "RTD-01 (ºC)"=w1603:sgl, "vacuo (mBar)"=w1604:dbl, "P02 (Bar)"=w1600:dbl, "RTD-chamber (ºC)"=w1601:sgl, "P01 (Bar)"=w1605:dbl, "32bytes"=w1606:bool)  [unwired: 5 in]
                            }
                            n971 = property on="Save Discharge" class="Bool (strict)"() -> ("Value"=w1583:bool)  [unwired: 2 in, 2 out]
                            n972 = case shown="True" w1583 {
                              frame False {
                              }
                              frame True {
                                n973 = property on="Cycles" class="DigNum (strict)"() -> ("Value"=w1597:dbl)  [unwired: 2 in, 2 out]
                                n974 = property on="Set ChM" class="DigNum (strict)"() -> ("Value"=w1596:dbl)  [unwired: 2 in, 2 out]
                                n975 = Increment(x=w1597) -> (x+1=w1598:dbl)
                                n976 = Increment(x=w1596) -> (x+1=w1599:dbl)
                                n977 = local write "Cycles"(w1598) -> ()
                                n978 = local write "Set ChM"(w1599) -> ()
                              }
                            }
                            n979 = Wait Until Next ms Multiple(millisecond multiple=u32 5) -> ()  [unwired: 1 out]
                            n980 = local write "Vol01"(w1594) -> ()
                            n981 = local write "Vol02"(w1591) -> ()
                            n982 = Multiply(x=w1590, y=0.001) -> (x*y=w1588:dbl)
                            n983 = local write "Pcin"(w1588) -> ()
                            n984 = Merge Signals(w1594, w1593, w1590, w1587, w1585, w1586, w1588) -> (w1592:dynamicdata)
                            n985 = local write "graph_completo"(w1592) -> ()
                            n986 = property on="Ch Max" class="Bool (strict)"() -> ("Value"=w1581:bool)  [unwired: 2 in, 2 out]
                            n987 = property on="ISO Start" class="Bool (strict)"() -> ("Value"=w1582:bool)  [unwired: 2 in, 2 out]
                            n988 = property on="V V Start" class="Bool (strict)"() -> ("Value"=w1580:bool)  [unwired: 2 in, 2 out]
                            n989 = And(x=w1580, y=w1581) -> (x .and. y?=w1579:bool)
                            n990 = And(x=w1579, y=w1582) -> (x .and. y?=w1578:bool)
                            n991 = Equal?(x=w1578, y=FALSE) -> (x = y?=w1576:bool)
                          }
                          frame #5 {
                            n992 = property on="ISO Start" class="Bool (strict)"() -> ("Value"=w1611:bool)  [unwired: 2 in, 2 out]
                            n993 = Not(x=w1609) -> (.not. x?=w1612:bool)
                            n994 = case shown="False" w1608 {
                              tunnel: w1609 -> [w1614 _]
                              tunnel: [FALSE ("write") TRUE ("write")] -> w1607
                              frame False {
                                n995 = local write "Charge"(w1614) -> ()
                              }
                              frame True {
                              }
                            }
                            n996 = local write "clear sample"(w1612) -> ()
                            n997 = local write "Discharge"(w1612) -> ()
                            n998 = case shown="True" w1611 {
                              tunnel: [FALSE ("write") TRUE ("write")] -> w1610
                              frame False {
                              }
                              frame True {
                              }
                            }
                          }
                        }
                        n999 = Or(x=w1548, y=w1546) -> (x .or. y?=w1547:bool)
                      }
                    }
                  }
                }
              }
            }
          }
        }
      }
    }
    n1000 = property class="Pnl"(reference=w57, error in=w56) -> (error out=w60:errorcluster, "Panes[]"=w58:refnum<vi>[])  [unwired: 1 out]
    n1001 = Not(x="stop") -> (.not. x?=→"Stop":bool)
    n1002 = Index Array(array=w58) -> (element=w59:refnum<vi>)  [unwired: 1 in]
    n1003 = property class="Pane"(reference=w59, error in=w60, "PaneColor"=u32 13626623 ("Color Box")) -> ()  [unwired: 2 out]
    n1004 = case shown="True" "close All" {
      selector: "close All" -> [_ w66]
      tunnel: [w63 w66] -> w49
      tunnel: "Vertical Pause Button" -> [w63 _]
      frame False {
      }
      frame True {
        n1005 = stacked-sequence {
          tunnel: 0.0 ("number") -> [w68 w72 w75 w79 w83]
          tunnel: TRUE ("write") -> [w67 w71 w76 w80 w84]
          frame #0 {
            n1006 = call "data2byte.vi"("argument"=w68, "new function"=1.0) -> ("protocol"=w69:string)  [unwired: 8 in, 1 out]
            n1007 = call "Advanced Serial.vi"("Write"=w67, "string to write"=w69) -> ()  [unwired: 3 in, 7 out]
          }
          frame #1 {
            n1008 = call "data2byte.vi"("argument"=w72, "new function"=2.0) -> ("protocol"=w73:string)  [unwired: 8 in, 1 out]
            n1009 = call "Advanced Serial.vi"("Write"=w71, "string to write"=w73) -> ()  [unwired: 3 in, 7 out]
          }
          frame #2 {
            n1010 = call "data2byte.vi"("argument"=w75, "new function"=3.0) -> ("protocol"=w77:string)  [unwired: 8 in, 1 out]
            n1011 = call "Advanced Serial.vi"("Write"=w76, "string to write"=w77) -> ()  [unwired: 3 in, 7 out]
          }
          frame #3 {
            n1012 = call "data2byte.vi"("argument"=w79, "new function"=4.0) -> ("protocol"=w81:string)  [unwired: 8 in, 1 out]
            n1013 = call "Advanced Serial.vi"("Write"=w80, "string to write"=w81) -> ()  [unwired: 3 in, 7 out]
          }
          frame #4 {
            n1014 = call "data2byte.vi"("argument"=w83, "new function"=5.0) -> ("protocol"=w85:string)  [unwired: 8 in, 1 out]
            n1015 = call "Advanced Serial.vi"("Write"=w84, "string to write"=w85) -> ()  [unwired: 3 in, 7 out]
          }
        }
      }
    }
    n1016 = case shown="True" w49 {
      tunnel: [FALSE ("stop 2") w62] -> w47
      frame False {
      }
      frame True {
        n1017 = call "SCC-manual.vi"() -> ("Boolean"=w62:bool)  [unwired: 11 out]
      }
    }
    n1018 = property on="close All" class="Bool (strict)"("Value"=w47) -> ()  [unwired: 2 in, 2 out]
    n1019 = property on="Vertical Pause Button" class="Bool (strict)"("Value"=w47) -> ()  [unwired: 2 in, 2 out]
    n1020 = Or(x=w45, y="stop") -> (x .or. y?=w46:bool)
  }
  n1021 = local write "Set ChM"(w8) -> ()
  n1022 = local write "Cycles"(w8) -> ()
  n1023 = local write "Cycles"(1.0 ("Cycles")) -> ()
  n1024 = local write "N 1bar"(0 ("N 1bar")) -> ()
  n1025 = local write "Set v v"(1.0 ("Set v v")) -> ()
  n1026 = local write "total Time(min)"(5.0 ("total Time(min)")) -> ()
  n1027 = local write "size(s)"(0 ("size(s)")) -> ()
  n1028 = local write "cargas-vol1"(0.0 ("cargas")) -> ()
  n1029 = local write "slope"(0.0 ("slope")) -> ()
  n1030 = local write "Ndata"(3 ("Ndata")) -> ()
  n1031 = local write "t-on"(0.0 ("%t-on")) -> ()
  n1032 = local write "PID limit 2"(2.0 ("PID limit")) -> ()
  n1033 = local write "time (s) Loop"(1.0 ("time PID")) -> ()
  n1034 = local write "X time Off"(1.0 ("X time Off")) -> ()
  n1035 = local write "time-loop"(1.0 ("time-loop")) -> ()
  n1036 = stacked-sequence {
    tunnel: 0.0 ("number") -> [w1771 w1775 w1778 w1782 w1786]
    tunnel: TRUE ("write") -> [w1770 w1774 w1779 w1783 w1787]
    frame #0 {
      n1037 = call "data2byte.vi"("argument"=w1771, "new function"=1.0) -> ("protocol"=w1772:string)  [unwired: 8 in, 1 out]
      n1038 = call "Advanced Serial.vi"("Write"=w1770, "string to write"=w1772) -> ()  [unwired: 3 in, 7 out]
    }
    frame #1 {
      n1039 = call "data2byte.vi"("argument"=w1775, "new function"=2.0) -> ("protocol"=w1776:string)  [unwired: 8 in, 1 out]
      n1040 = call "Advanced Serial.vi"("Write"=w1774, "string to write"=w1776) -> ()  [unwired: 3 in, 7 out]
    }
    frame #2 {
      n1041 = call "data2byte.vi"("argument"=w1778, "new function"=3.0) -> ("protocol"=w1780:string)  [unwired: 8 in, 1 out]
      n1042 = call "Advanced Serial.vi"("Write"=w1779, "string to write"=w1780) -> ()  [unwired: 3 in, 7 out]
    }
    frame #3 {
      n1043 = call "data2byte.vi"("argument"=w1782, "new function"=4.0) -> ("protocol"=w1784:string)  [unwired: 8 in, 1 out]
      n1044 = call "Advanced Serial.vi"("Write"=w1783, "string to write"=w1784) -> ()  [unwired: 3 in, 7 out]
    }
    frame #4 {
      n1045 = call "data2byte.vi"("argument"=w1786, "new function"=5.0) -> ("protocol"=w1788:string)  [unwired: 8 in, 1 out]
      n1046 = call "Advanced Serial.vi"("Write"=w1787, "string to write"=w1788) -> ()  [unwired: 3 in, 7 out]
    }
  }
  n1047 = local write "PCS"(w1) -> ()
  n1048 = local write "T Ctrl"(w1) -> ()
  n1049 = local write "Charge"(w1) -> ()
  n1050 = local write "Discharge"(w1) -> ()
  n1051 = local write "close All"(w1) -> ()
  n1052 = local write "V V Start"(w1) -> ()
  n1053 = local write "Ch Max"(w1) -> ()
  n1054 = local write "ISO Start"(w1) -> ()
  n1055 = local write "Kinetic Save"(TRUE ("Kinetic Save")) -> ()
  n1056 = local write "descarga 2"(FALSE ("descarga")) -> ()
  n1057 = local write "N cycles"(10.0 ("N cycles")) -> ()
  n1058 = local write "Pressure Max"(10.0 ("Pressure Max")) -> ()
  n1059 = local write "t-vacuo (s) clean"(60.0 ("t-vacuo (s) clean")) -> ()
  n1060 = local write "Npoint"(20 ("Npoint")) -> ()
  n1061 = local write "Pmax"(10 ("Pmax")) -> ()
  n1062 = local write "dp/dt min"(0.1 ("dp/dt min")) -> ()
  n1063 = local write "Kp"(0.6 ("Kp")) -> ()
  n1064 = local write "Ki(s)"(0.5 ("Ki(s)")) -> ()
  n1065 = local write "fator Ganho"(100.0 ("y")) -> ()
  n1066 = local write "t-vacuo (s)"(120.0 ("t-vacuo (s)")) -> ()
  n1067 = local write "Mininum Slope"(1e-05 ("Min Slope")) -> ()
  n1068 = local write "Kd(s)"(0.125 ("Kd(s)")) -> ()
  n1069 = local write "command"("Start" ("command")) -> ()
  n1070 = local write "tempo"(dbl[] [] ("tempo")) -> ()
  n1071 = local write "cont_desc"(dbl[] [] ("output array 2")) -> ()
  n1072 = local write "time 2"(dbl[] [] ("output array 2")) -> ()
  n1073 = local write "Pvol2"(dbl[] [] ("output array 2")) -> ()
  n1074 = local write "cont_desc min"(dbl[] [] ("output array 2")) -> ()
  n1075 = local write "cont_vacuo"(u32[] [] ("output array 2")) -> ()
  n1076 = local write "array"(dbl[] [0.5, 1.0, 1.5, 2.0, 3.0, 5.0, 5.0, 5.0, 5.0, 7.0, 14.0, 18.0, 19.0, 20.0] ("array")) -> ()
  n1077 = local write "path"(path "H:/PCS-control/iso.txt" ("path")) -> ()
  n1078 = local write "pathVV"(path "H:/PCS-control/iso_vv.txt" ("path")) -> ()
  n1079 = local write "pathISO"(path "H:/PCS-control/iso_iso.txt" ("path")) -> ()
